vi "Product Romete Exchange.vi"(8 "error in (no error)":errorcluster, 11 "Main":T1={"Tite"="", "Base path"=path "", "Table"=[], "Stations"=[], "Shield Array"=[], "UPHs"=[], "VISA"={"VISA"="", "baud rate"=9600, "data bits"=8, "parity"=enum."None", "stop bits"=10, "flow control"=0}, "Path"={"roof"=path "", "Config"=path "", "Png"=path ""}, "Ctr"={"DB Dispaly"=refnum, "Error Table"=refnum, "Display"=refnum, "Login"=refnum, "Exit"=refnum, "FTT_Submit"=refnum}, "Login"={"User"="", "Grade"=""}, "information"={"cause"="", "Type"=enum."Inform", "code"=0, "Suroce"="", "Status"=FALSE}, "Local DB"={"Connstr"="", "Database"={"Constr"={"Driver"="", "Server"="", "User"="", "Pwd"="", "Database"=""}, "conn ref"=refnum, "State"=FALSE}}, "Remote DB"={"Connstr"="", "Database"={"Constr"={"Driver"="", "Server"="", "User"="", "Pwd"="", "Database"=""}, "conn ref"=refnum, "State"=FALSE}}, "FTT TV"="", "ExchangeTime"=0, "NVH"="", "EOL Path"=path ""} {"VISA"."flow control" items=["None", "XON/XOFF", "RTS/CTS", "XON/XOFF & RTS/CTS", "DTR/DSR", "XON/XOFF & DTR/DSR"]; "VISA"."stop bits" items=["1.0"=10, "1.5"=15, "2.0"=20]}) -> (0 "error out":errorcluster)   [LabVIEW 2014]
uses:
  <vilib>/addons/database/_DB Variant To Data/Database Variant To Data.xnode
  Type'def/AJ_RunTable.ctl
  Type'def/Exchange Table.ctl
  <vilib>/ptbypt/NI_PtbyPt.lvlib
  Simatic S7/Function/Read/Read Sigle Data/Read Sigle String.vi
  <vilib>/addons/database/NI_Database_API.lvlib
  Type'def/BR Exchange(Romte).ctl
  Type'def/Online_Table.ctl
  Simatic S7/Function/Write/Write Sigle Data/Write Sigle Bool.vi
  Type'def/UPH Config.ctl
  VISA/Ctr/VISA Ctr.ctl
  Type'def/Main Ctr Ref.ctl
  Type'def/User Login.ctl
  Database/Ctr/Constr.ctl
  <vilib>/addons/database/Connection.llb/Conn ObjectReference.ctl
  Database/Ctr/Conneect State.ctl
  Type'def/MainCtr.ctl
panel:
  out "Previous Event":string
  in  "Test":bool
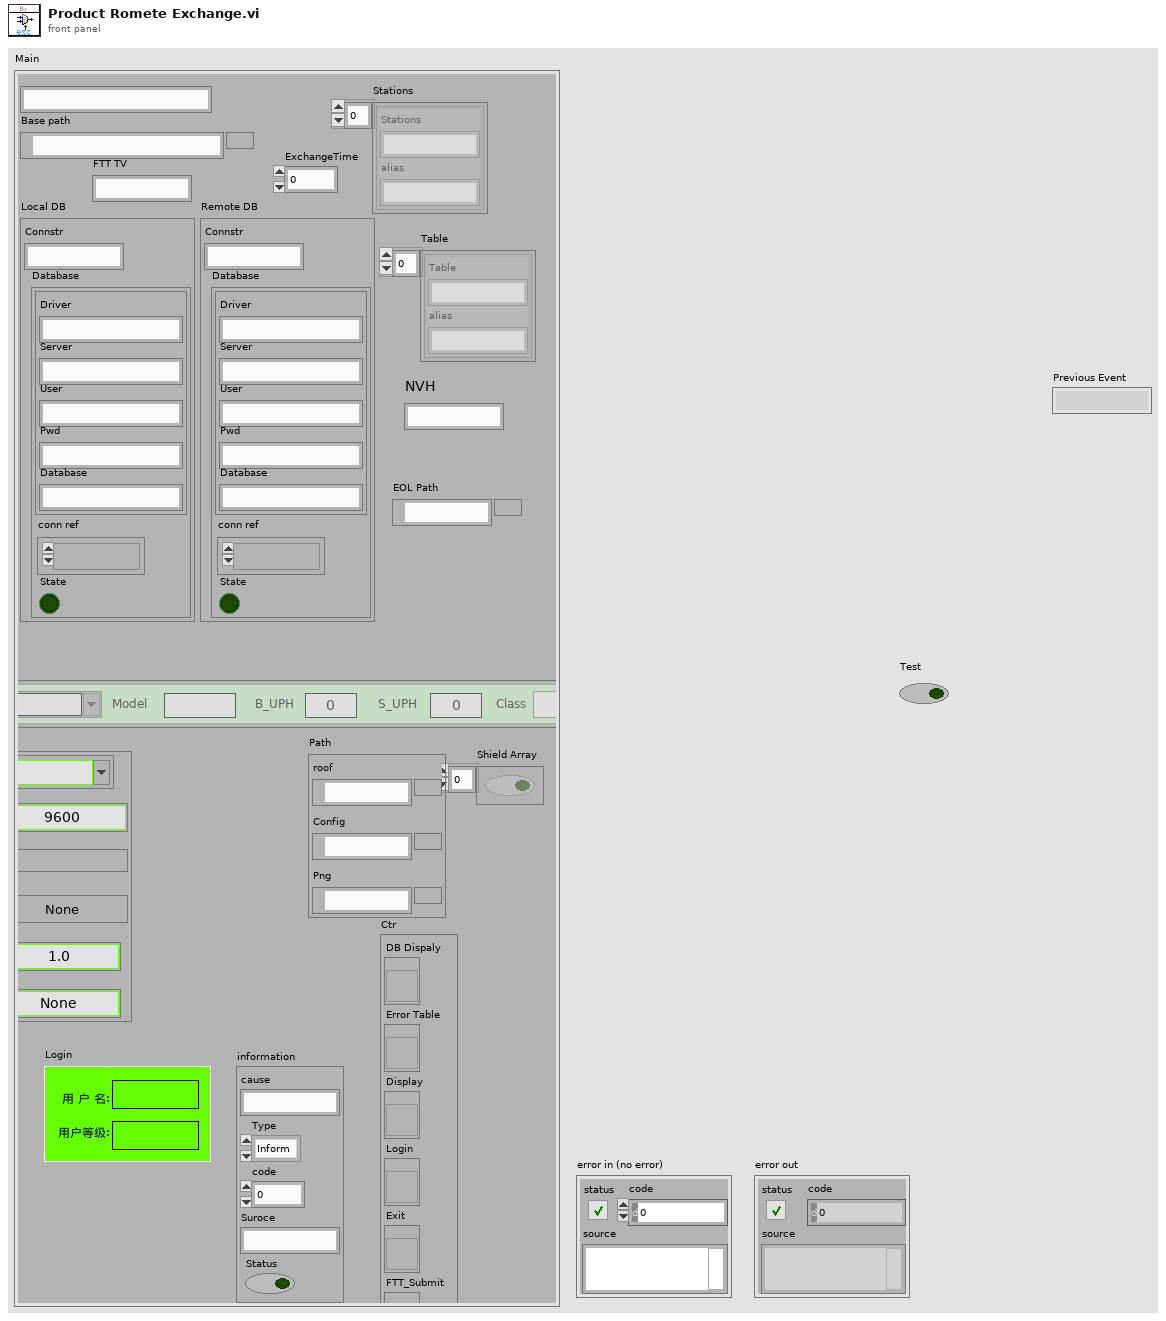
[diagram p1: front panel]
types:
  T1 = typedef "MainCtr.ctl" = cluster{"Tite":string, "Base path":path, "Table":cluster{"Table":string, "alias":string}[], "Stations":cluster{"Stations":string, "alias":string}[], "Shield Array":bool[], "UPHs":T2[], "VISA":T3, "Path":cluster{"roof":path, "Config":path, "Png":path}, "Ctr":T4, "Login":T5, "information":cluster{"cause":string, "Type":enum16{"Inform", "Warning", "Alarm"}, "code":i32, "Suroce":string, "Status":bool}, "Local DB":cluster{"Connstr":string, "Database":T6}, "Remote DB":cluster{"Connstr":string, "Database":T6}, "FTT TV":string, "ExchangeTime":i32, "NVH":string, "EOL Path":path}
  T2 = typedef "UPH Config.ctl" = cluster{"Line_No":string, "Model":string, "B_UPH ":i16, "S_UPH  ":i16, "Class":enum16{"Big", "Small"}}
  T3 = typedef "VISA Ctr.ctl" = cluster{"VISA":refnum<visa-resource-name>, "baud rate":u32, "data bits":u16, "parity":enum16{"None", "Odd", "Even", "Mark", "Space"}, "stop bits":u16, "flow control":u16}
  T4 = typedef "Main Ctr Ref.ctl" = cluster{"DB Dispaly":refnum<vi>, "Error Table":refnum<vi>, "Display":refnum<vi>, "Login":refnum<vi>, "Exit":refnum<vi>, "FTT_Submit":refnum<vi>}
  T5 = typedef "User Login.ctl" = cluster{"User":string, "Grade":string}
  T6 = typedef "Conneect State.ctl" = cluster{"Constr":T7, "conn ref":T8, "State":bool}
  T7 = typedef "Constr.ctl" = cluster{"Driver":string, "Server":string, "User":string, "Pwd":string, "Database":string}
  T8 = typedef "NI_Database_API.lvlib/Conn ObjectReference.ctl" = refnum<k1>
  T9 = cluster{"Next PN":cluster{"SN":string, "Model":string, "Pos":i32}, "PrePN":cluster{"SN":string, "Model":string, "Pos":i32}}
  T10 = typedef "Exchange Table.ctl" = cluster{"LineName":string, "Model":string, "Station":string, "StartTime":timestamp, "EndTime":timestamp, "SubTime":dbl}
  T11 = typedef "AJ_RunTable.ctl" = cluster{"LineName":string, "ProjectName":string, "AcutalOuput":u32, "ProStatus":string, "PlanOutput":u32, "ProTime":u32, "ShiftFlag":string}
  T12 = cluster{"cause":string, "Type":enum16{"Inform", "Warning", "Alarm"}, "code":i32, "Suroce":string, "Status":bool}
  T13 = typedef "BR Exchange(Romte).ctl" = cluster{"Line Name":string, "Start Tine":timestamp, "End Time":timestamp, "PrePN":string, "NextPN":string, "Status":bool}
  T14 = cluster{"excT":dbl, "Pos":cluster{"Pre Pos":i32, "Next Pos":i32}, "relative s":dbl, "Exchange Table":T10, "Main ":T1, "BR":T13, "information":cluster{"cause":string, "Type":enum16{"Inform", "Warning", "Alarm"}, "code":i32, "Suroce":string, "Status":bool}, "UPH Model":string[], "FTT Log":string[], "AJ Run":T11, "Exc flag":cluster{"Exchange Enable":bool, "ms":dbl}, "ExcPN":cluster{"Next PN":cluster{"SN":string, "Model":string, "Pos":i32}, "PrePN":cluster{"SN":string, "Model":string, "Pos":i32}}}
  T15 = typedef "Online_Table.ctl" = cluster{"SN":string, "Frame":string, "Station":string, "Model":string, "Color":string, "OnTime":timestamp, "OutTime":timestamp, "Repaired":i32, "OnRepair":bool, "Pstate":string}
  T16 = cluster{"Array str[0]":string, "Array str[1]":string, "Array str[2]":string, "Array str[3]":string, "Array str[4]":string, "Array str[5]":string, "Array str[6]":string, "Array str[7]":string, "Array str[8]":string, "Array str[9]":string, "Array str[10]":string}
  T17 = typedef "FTT Display Type.ctl" = cluster{"Line.No":string, "Model":string, "Color":string, "UPH":dbl, "Plan":dbl, "Target Rate":dbl, "Target ":dbl, "Actual":dbl, "FTT":dbl, "FTT Rate":dbl, "Repaired":dbl, "Reject":dbl, "Ouline":dbl, "Line State":string}
  T18 = cluster{"Display":T17, "Class":enum16{"Big", "Small"}}
  T19 = typedef "Phone Var.ctl" = cluster{"Mes":bool, "Model":string}
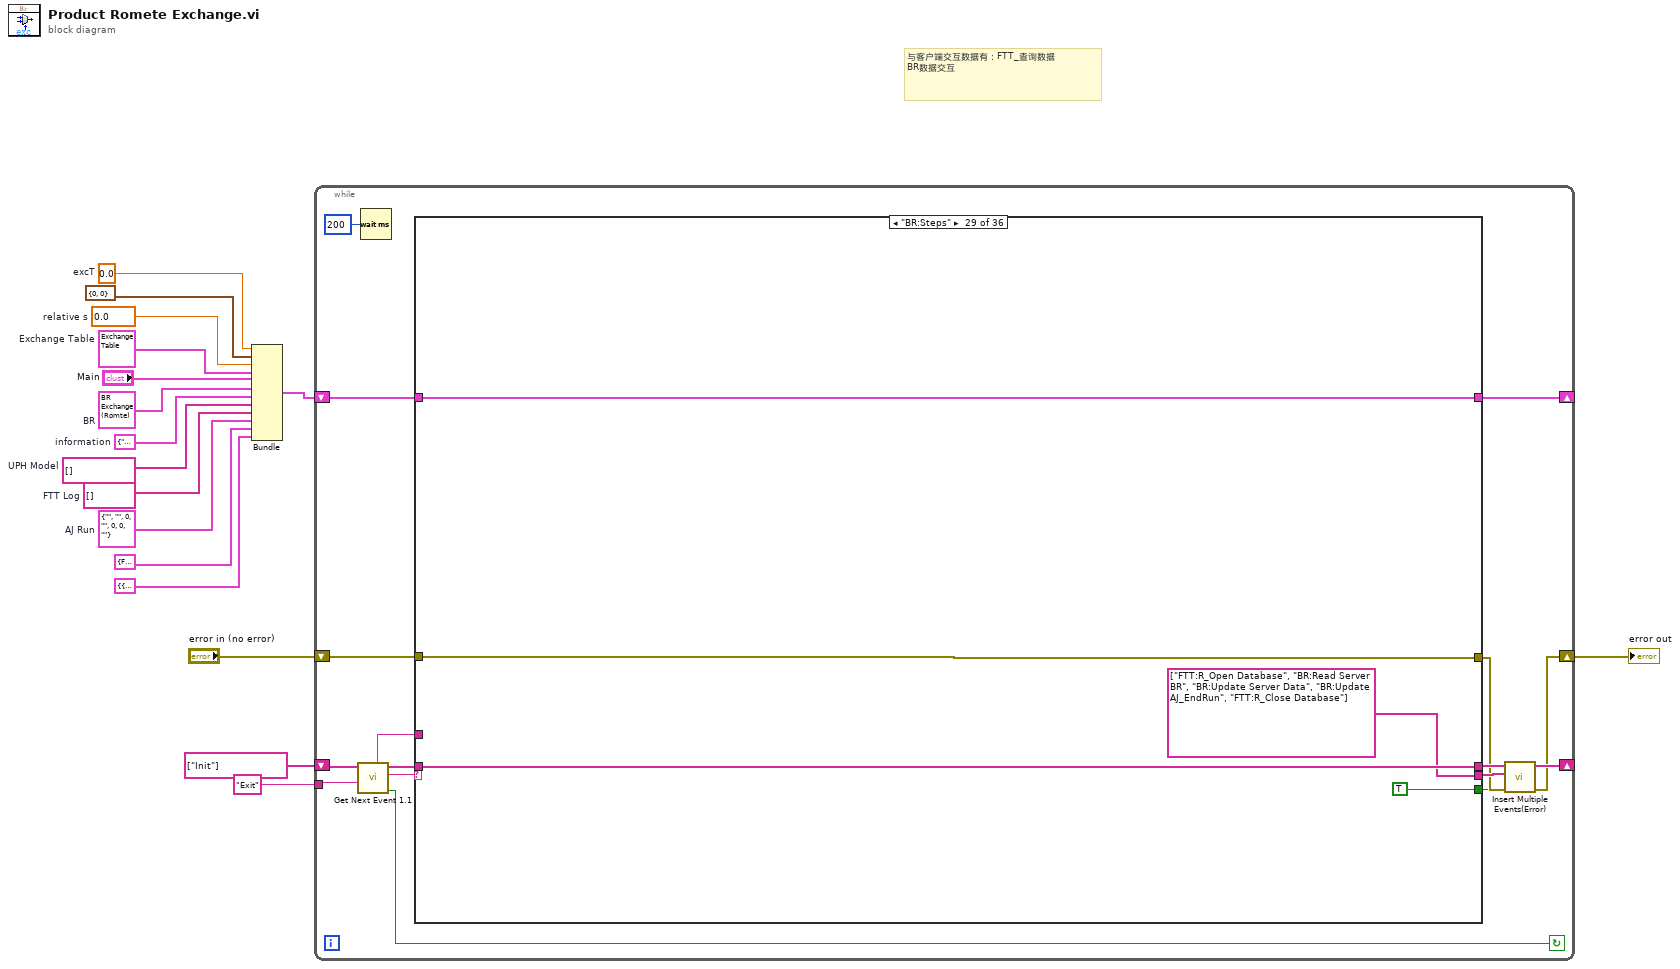
[diagram p0: block diagram]
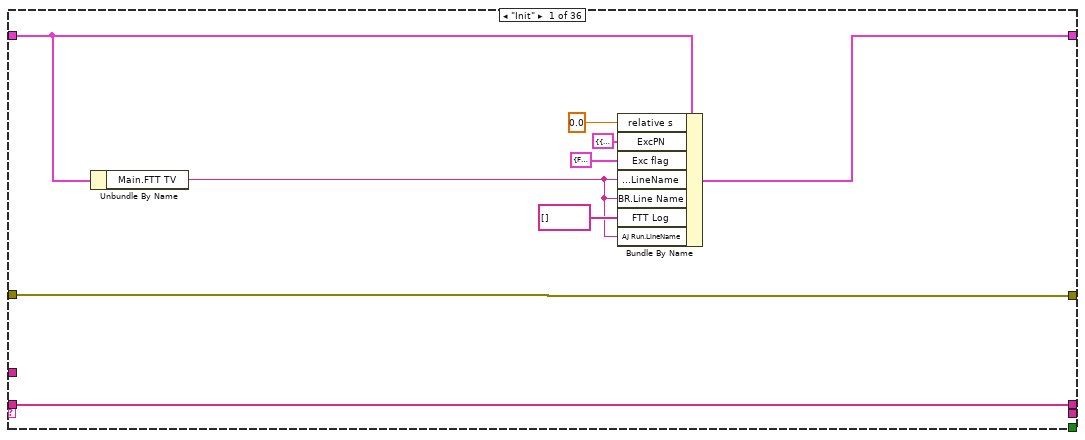
[diagram p2: hidden frame]
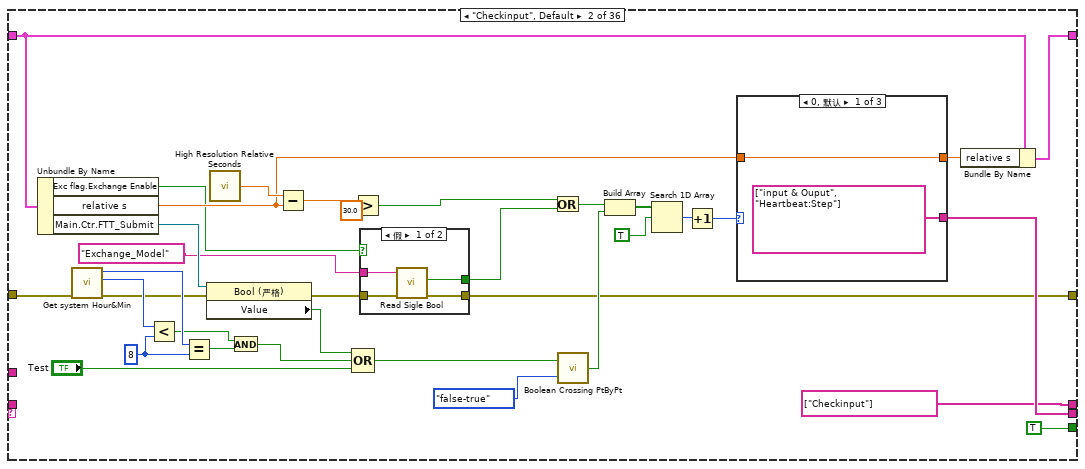
[diagram p3: hidden frame]
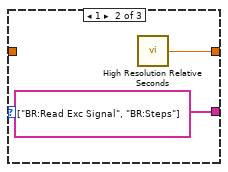
[diagram p5: hidden frame]
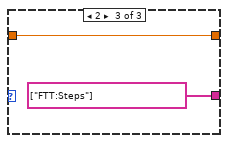
[diagram p6: hidden frame]
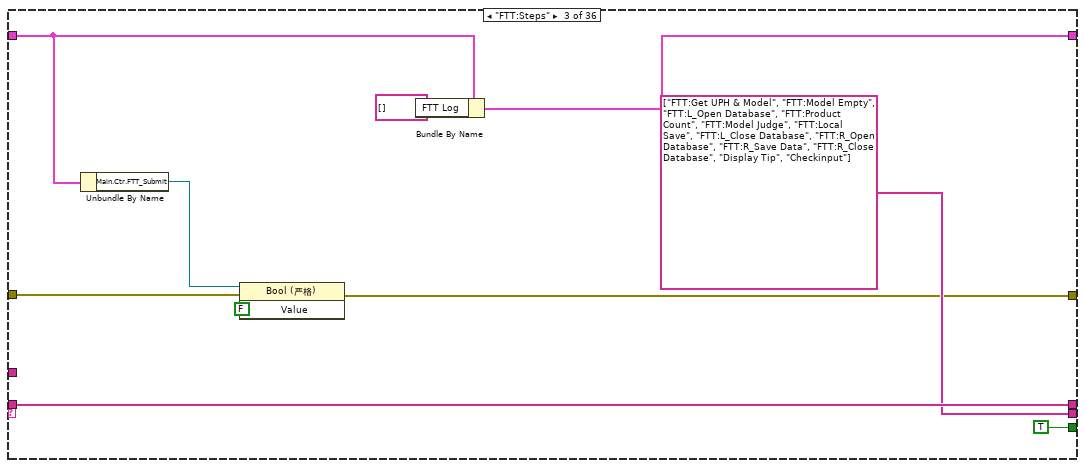
[diagram p7: hidden frame]
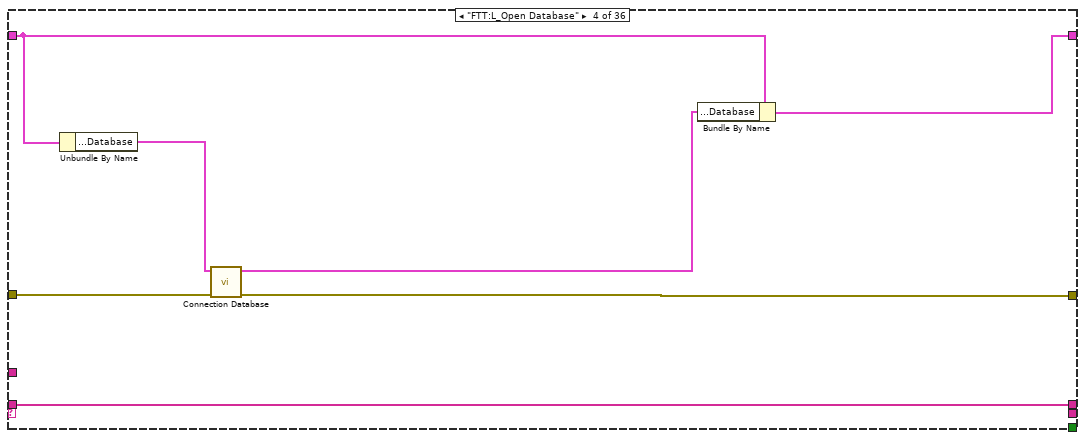
[diagram p8: hidden frame]
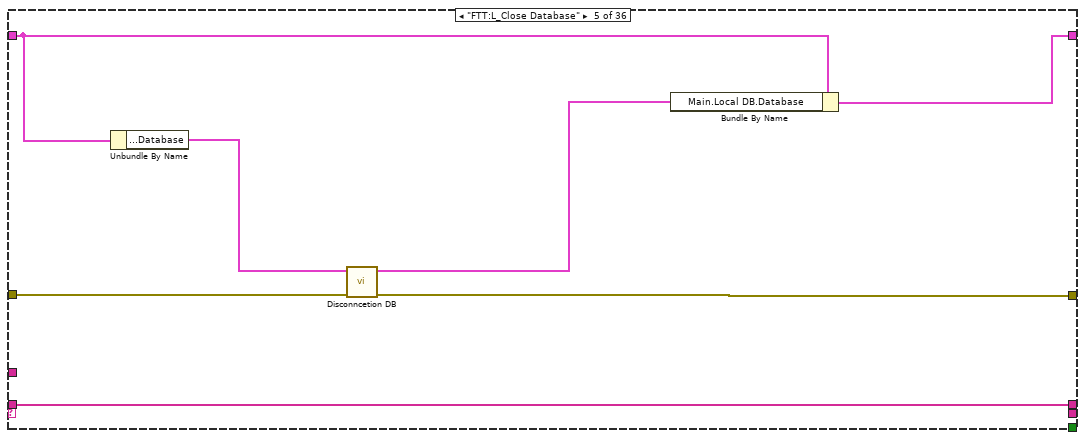
[diagram p9: hidden frame]
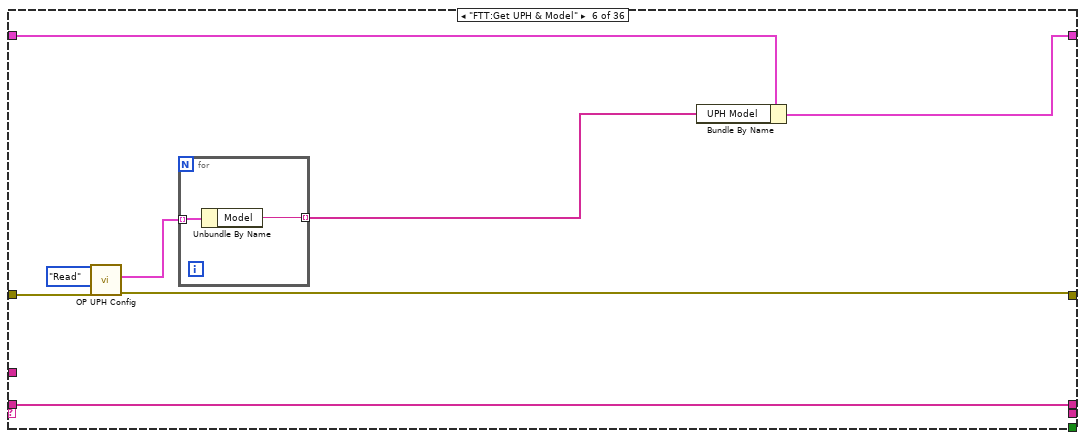
[diagram p10: hidden frame]
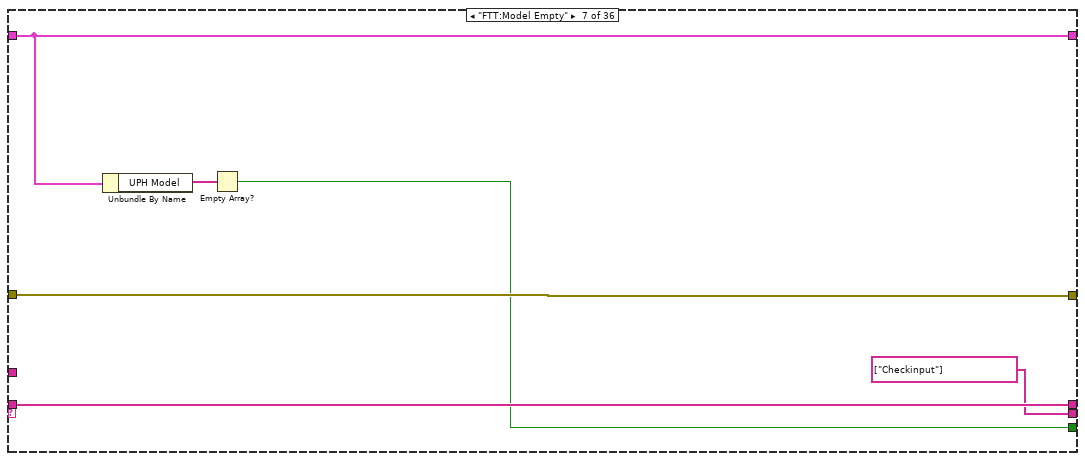
[diagram p11: hidden frame]
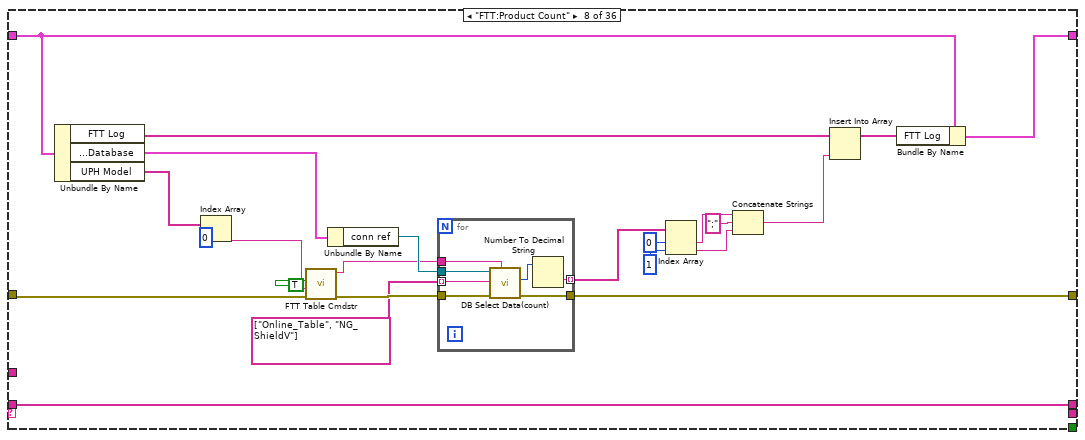
[diagram p12: hidden frame]
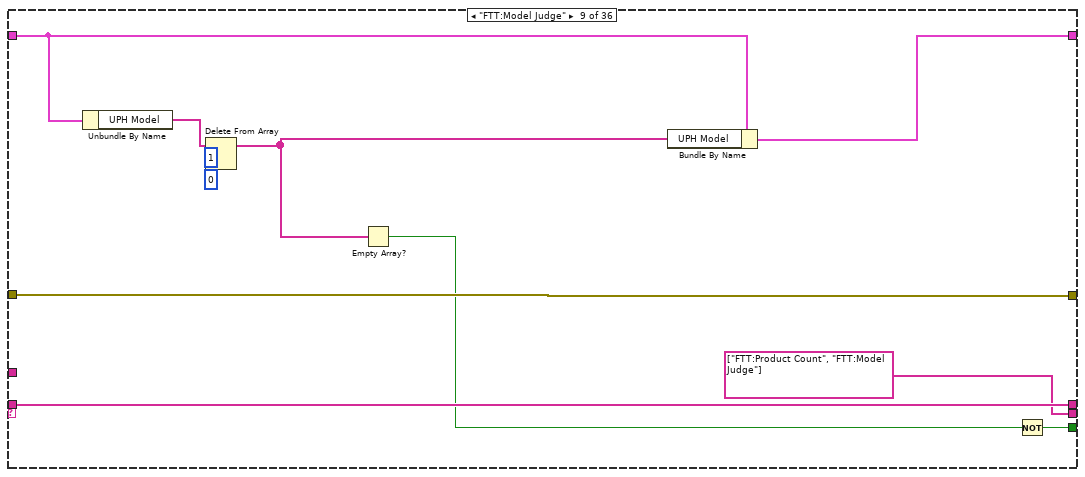
[diagram p13: hidden frame]
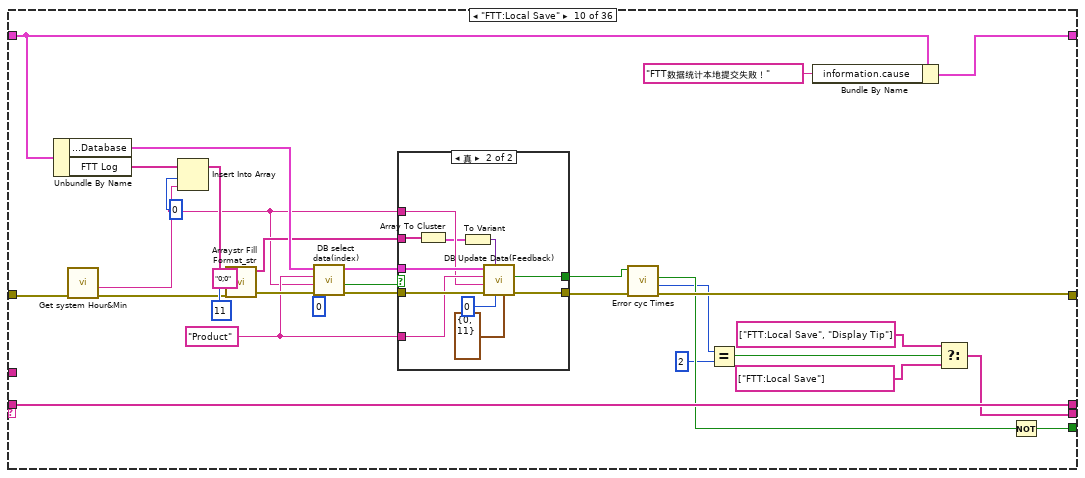
[diagram p14: hidden frame]
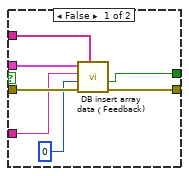
[diagram p15: hidden frame]
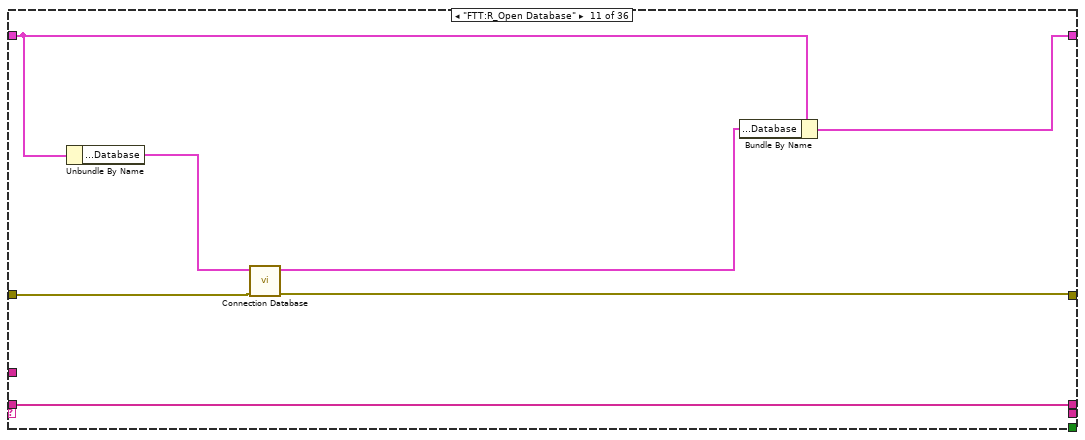
[diagram p16: hidden frame]
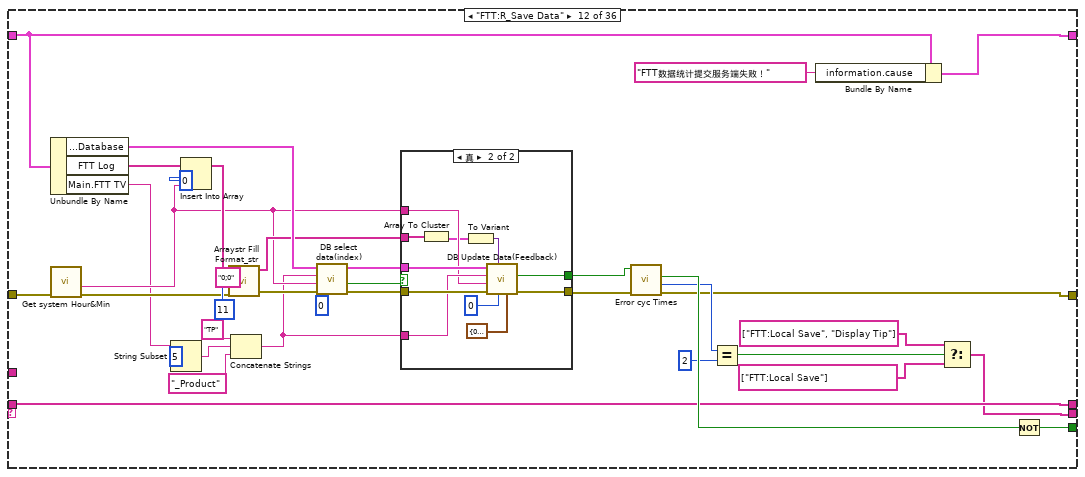
[diagram p17: hidden frame]
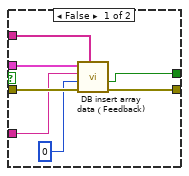
[diagram p18: hidden frame]
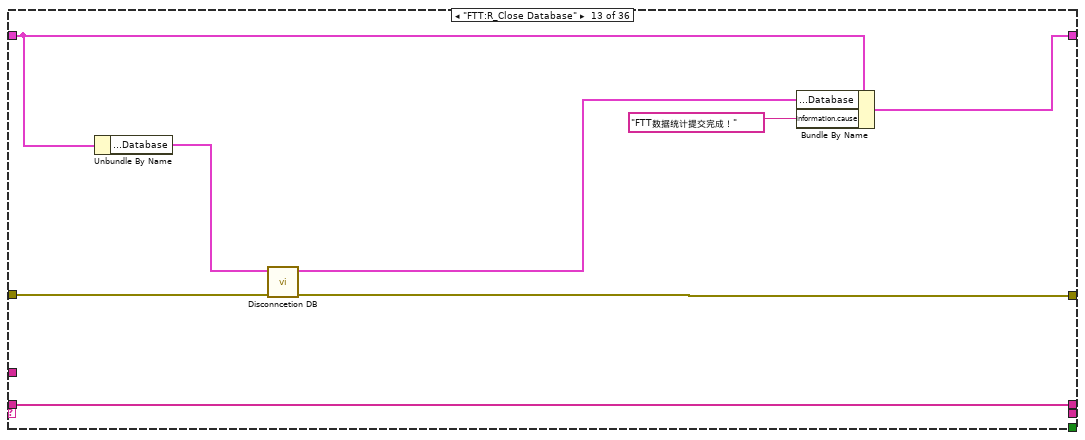
[diagram p19: hidden frame]
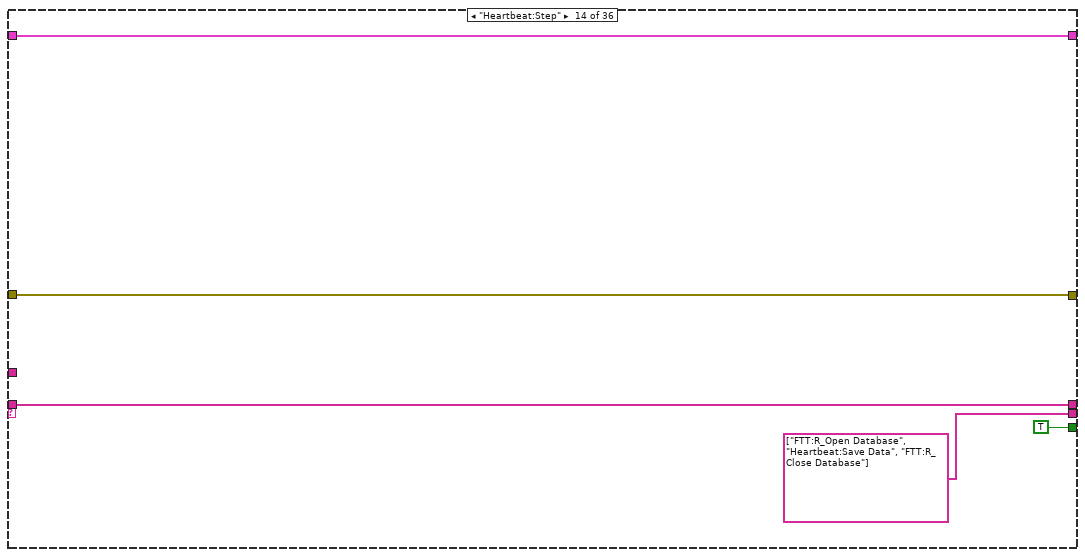
[diagram p20: hidden frame]
diagram:
  w1 = 0.0  # excT
  w3 = 0.0  # relative s
  w6 = T10 {"LineName"="", "Model"="", "Station"="", "StartTime"=timestamp(0 s since 1904-01-01), "EndTime"=timestamp(0 s since 1904-01-01), "SubTime"=0.0}  # Exchange Table
  w7 = T11 {"LineName"="", "ProjectName"="", "AcutalOuput"=0, "ProStatus"="", "PlanOutput"=0, "ProTime"=0, "ShiftFlag"=""}  # AJ Run
  w8 = string[] []  # FTT Log
  w9 = string[] []  # UPH Model
  w10 = T12 {"cause"="", "Type"=enum."Inform", "code"=0, "Suroce"="", "Status"=FALSE}  # information
  w12 = T13 {"Line Name"="", "Start Tine"=timestamp(0 s since 1904-01-01), "End Time"=timestamp(0 s since 1904-01-01), "PrePN"="", "NextPN"="", "Status"=FALSE}  # BR
  # "与客户端交互数据有：FTT_查询数据\nBR数据交互"
  n1 = Bundle("excT"=w1, "Pos"=cluster{"Pre Pos":i32, "Next Pos":i32} {"Pre Pos"=0, "Next Pos"=0}, "relative s"=w3, "Exchange Table"=w6, "Main"="Main", "BR"=w12, "information"=w10, "UPH Model"=w9, "FTT Log"=w8, "AJ Run"=w7, "Exc flag"=cluster{"Exchange Enable":bool, "ms":dbl} {"Exchange Enable"=FALSE, "ms"=0.0}, "ExcPN"=T9 {"Next PN"={"SN"="", "Model"="", "Pos"=0}, "PrePN"={"SN"="", "Model"="", "Pos"=0}}) -> (w14:T14)  [unwired: 1 in]
  n2 = while {
    tunnel: "Exit" ("Exit Event") -> [w30]
    shift-right: [w26] -> _
    shift-left: string[] ["Init"] -> [w31]
    shift-right: [w21] -> w11
    shift-left: "error in (no error)" -> [w29]
    shift-right: [w23] -> _
    shift-left: w14 -> [w27]
    stop <- w32 continue-if-true
    n3 = call "Get Next Event 1.1.vi"("Exit Event"=w30, "event queue in"=w31) -> ("Condition (Exit:F)"=w32:bool, "next event"=w33:string, "event queue out"=w28:string[], "Previous Event"=w18:string)  [unwired: 6 in]
    n4 = Wait (ms)(milliseconds to wait=u32 200) -> ()  [unwired: 1 out]
    n5 = case shown="\"BR:Steps\"" w33 {
      tunnel: w29 -> [w41 w76 w95 w105 w111 w120 w126 w151 w166 w195 w225 w233 w286 w291 w317 w354 w359 w364 w377 w404 w457 w860 w919 w983 w1254 w1305 w1712 w2017 w2066 w2079 w2343 w2399 w2468 w2474 w2479 w2490]
      tunnel: w28 -> [w42 _ w98 w104 w112 w113 w125 w140 w165 w179 w224 w238 w287 w290 w314 w355 w358 w362 w374 w403 w458 w861 w920 w979 w1255 w1277 w1706 w2006 w2065 w2069 w2338 w2404 w2464 w2470 w2478 _]
      tunnel: w27 -> [w36 w55 w90 w102 w108 w116 w128 w130 w160 w181 w221 w234 w284 w292 w295 w348 w360 w367 w370 w401 w455 w853 w903 w959 w1243 w1286 w1701 w1997 w2067 w2072 w2325 w2403 w2466 w2475 w2480 w2487]
      tunnel: [w41 w46 w93 w99 w109 w118 w126 w141 w166 w182 w222 w235 w282 w291 w304 w353 w359 w364 w375 w399 w456 w859 w900 w969 w1250 w1288 w1702 w1994 w2066 w2070 w2334 w2402 w2467 w2472 w2479 w2488] -> w22
      tunnel: [w42 string[] ["Checkinput"] w98 w104 w112 w113 w125 w140 w165 w179 w224 w238 w287 w290 w314 w355 w358 w362 w374 w403 w458 w861 w920 w979 w1255 w1277 w1706 w2006 w2065 w2069 w2338 w2404 w2464 w2470 w2478 string[] ["Checkinput"]] -> w25
      tunnel: [_ TRUE ("Insert all? (T)") TRUE ("Insert all? (T)") _ _ _ w124 _ w164 w178 _ w236 _ TRUE ("Insert all? (T)") w303 TRUE ("Insert all? (T)") TRUE ("Insert all? (T)") w363 _ _ _ _ w910 w965 w1244 _ w1698 w2005 TRUE ("Insert all? (T)") _ w2333 w2401 _ w2471 TRUE ("Insert all? (T)") FALSE ("Insert all? (T)")] -> w20
      tunnel: [_ w68 string[] ["FTT:Get UPH & Model", "FTT:Model Empty", "FTT:L_Open Database", "FTT:Product Count", "FTT:Model Judge", "FTT:Local Save", "FTT:L_Close Database", "FTT:R_Open Database", "FTT:R_Save Data", "FTT:R_Close Database", "Display Tip", "Checkinput"] _ _ _ string[] ["Checkinput"] _ string[] ["FTT:Product Count", "FTT:Model Judge"] w172 _ w237 _ string[] ["FTT:R_Open Database", "Heartbeat:Save Data", "FTT:R_Close Database"] w298 w342 string[] ["FTT:L_Open Database", "Exchange:Init Steps", "Exchange:Get Next SN", "Exchange:Serch SN Pos", "Exchange:Exc PrePN Table", "Exchange:Exc NextPN Table Update", "Exchange:End Judge", "FTT:L_Close Database"] string[] ["Exchange:Ready ok", "Exchange:Reset Exc Signal", "Display Tip"] _ _ _ _ w906 w972 string[] ["Exchange:Read OutTime", "Exchange:Get Esc SubTimeMax", "Display Tip"] _ string[] ["Display Tip", "FTT:R_Open Database", "Exchange:Server_exc Table", "FTT:R_Close Database"] w2000 string[] ["FTT:R_Open Database", "BR:Read Server BR", "BR:Update Server Data", "BR:Update AJ_EndRun", "FTT:R_Close Database"] _ w2326 w2400 _ string[] ["Quit"] string[] ["Exit"] _] -> w24
      tunnel: [w39 w54 w89 w101 w106 w115 w128 w129 w159 w180 w220 w232 w283 w292 w294 w347 w360 w367 w369 w400 w454 w852 w902 w958 w1243 w1285 w1700 w1996 w2067 w2071 w2325 w2403 w2466 w2475 w2480 w2487] -> w23
      tunnel: w18 -> [_ _ _ _ _ _ _ _ _ _ _ _ _ _ _ _ _ _ _ _ _ _ _ _ _ _ _ _ _ _ _ _ _ _ _ w2482]
      frame "Init" {
        n6 = Unbundle By Name(w36) -> ("Main.FTT TV"=w34:string)
        n7 = Bundle By Name(cluster=w36, "relative s"=0.0, "ExcPN"=T9 {"Next PN"={"SN"="", "Model"="", "Pos"=0}, "PrePN"={"SN"="", "Model"="", "Pos"=0}}, "Exc flag"=cluster{"Exchange Enable":bool, "ms":dbl} {"Exchange Enable"=FALSE, "ms"=0.0}, "Exchange Table.LineName"=w34, "BR.Line Name"=w34, "FTT Log"=string[] [], "AJ Run.LineName"=w34) -> (w39:T14)
      }
      frame "Checkinput", Default {
        w73 = 8 ("hour")
        n8 = Unbundle By Name(w55) -> ("Exc flag.Exchange Enable"=w48:bool, "relative s"=w53:dbl, "Main.Ctr.FTT_Submit"=w65:refnum<vi>)
        n9 = call "Get system Hour&Min.vi"("error in (no error)"=w76) -> ("error out"=w66:errorcluster, "minute"=w74:i32, "hour"=w75:i32)  [unwired: 7 in, 1 out]
        n10 = Less?(x=w74, y=w73) -> (x < y?=w71:bool)
        n11 = Equal?(x=w75, y=w73) -> (x = y?=w72:bool)
        n12 = property class="Bool (严格)"(reference=w65, error in=w66) -> (error out=w49:errorcluster, "Value"=w64:bool)  [unwired: 1 out]
        n13 = call <vilib>:"High Resolution Relative Seconds.vi"() -> ("relative seconds"=w63:dbl)
        n14 = And(x=w71, y=w72) -> (x .and. y?=w69:bool)
        n15 = Subtract(x=w63, y=w53) -> (x-y=w62:dbl)
        n16 = Compound Arithmetic op=OR(w64, w69, "Test") -> (w51:bool)
        n17 = Greater?(x=w62, y=30.0) -> (0:w44:bool)
        n18 = case shown="假" w48 {
          tunnel: w49 -> [w81 w82]
          tunnel: "Exchange_Model" ("Tags") -> [w80 _]
          tunnel: [w79 w82] -> w46
          tunnel: [w78 _] -> w43
          frame False {
            n19 = call "Read Sigle Bool.vi"("error in (no error)"=w81, "Tags"=w80) -> ("error out"=w79:errorcluster, "Boolean"=w78:bool)  [unwired: 7 in, 1 out]
          }
          frame True {
          }
        }
        n20 = Or(x=w44, y=w43) -> (x .or. y?=w45:bool)
        n21 = call <vilib>:"Boolean Crossing PtByPt.vi"("direction"=enum16{"either", "false-true", "true-false"}."false-true", "input"=w51) -> ("crossing"=w52:bool)  [unwired: 1 in]
        n22 = Build Array(w45, w52) -> (w60:bool[])
        n23 = Search 1D Array(1D array=w60, element=TRUE) -> (index of element=w58:i32)  [unwired: 1 in]
        n24 = Increment(x=w58) -> (x+1=w57:i32)
        n25 = case shown="0, 默认" w57 {
          tunnel: [string[] ["input & Ouput", "Heartbeat:Step"] string[] ["BR:Read Exc Signal", "BR:Steps"] string[] ["FTT:Steps"]] -> w68
          tunnel: [w83 w86 w87] -> w56
          tunnel: w53 -> [w83 _ w87]
          frame 0, Default {
          }
          frame 1 {
            n26 = call <vilib>:"High Resolution Relative Seconds.vi"() -> ("relative seconds"=w86:dbl)
          }
          frame 2 {
          }
        }
        n27 = Bundle By Name(cluster=w55, "relative s"=w56) -> (w54:T14)
      }
      frame "FTT:Steps" {
        n28 = Unbundle By Name(w90) -> ("Main.Ctr.FTT_Submit"=w94:refnum<vi>)
        n29 = property class="Bool (严格)"(reference=w94, error in=w95, "Value"=FALSE) -> (error out=w93:errorcluster)  [unwired: 1 out]
        n30 = Bundle By Name(cluster=w90, "FTT Log"=string[] []) -> (w89:T14)
      }
      frame "FTT:L_Open Database" {
        n31 = Unbundle By Name(w102) -> ("Main.Local DB.Database"=w103:T6)
        n32 = call "Connection Database.vi"("error in (no error)"=w105, "Connncet State"=w103) -> ("error out"=w99:errorcluster, "Connncet State out"=w100:T6)  [unwired: 8 in]
        n33 = Bundle By Name(cluster=w102, "Main.Local DB.Database"=w100) -> (w101:T14)
      }
      frame "FTT:L_Close Database" {
        n34 = Unbundle By Name(w108) -> ("Main.Local DB.Database"=w110:T6)
        n35 = call "Disconncetion DB.vi"("error in (no error)"=w111, "Connncet State"=w110) -> ("error out"=w109:errorcluster, "Connect State"=w107:T6)  [unwired: 8 in]
        n36 = Bundle By Name(cluster=w108, "Main.Local DB.Database"=w107) -> (w106:T14)
      }
      frame "FTT:Get UPH & Model" {
        n37 = call "OP UPH Config.vi"("error in (no error)"=w120, "Enum"=enum16{"init", "Read", "Write"}."Read") -> ("error out"=w118:errorcluster, "UPH out"=w117:T2[])  [unwired: 7 in, 1 out]
        n38 = for {
          tunnel: w117 -> [w122] mode=indexing
          tunnel: [w121] -> w114 mode=indexing
          n39 = Unbundle By Name(w122) -> ("Model"=w121:string)
        }
        n40 = Bundle By Name(cluster=w116, "UPH Model"=w114) -> (w115:T14)
      }
      frame "FTT:Model Empty" {
        n41 = Unbundle By Name(w128) -> ("UPH Model"=w127:string[])
        n42 = Empty Array?(array=w127) -> (empty?=w124:bool)
      }
      frame "FTT:Product Count" {
        n43 = Unbundle By Name(w130) -> ("FTT Log"=w133:string[], "Main.Local DB.Database"=w145:T6, "UPH Model"=w149:string[])
        n44 = Index Array(array=w149, index=0) -> (element=w148:string)
        n45 = call "FTT Table Cmdstr.vi"("error in (no error)"=w151, "Model"=w148, "Pstate"=TRUE) -> ("error out"=w146:errorcluster, "Str"=w143:string)  [unwired: 7 in]
        n46 = Unbundle By Name(w145) -> ("conn ref"=w144:T8)
        n47 = for {
          tunnel: w146 -> [w158]
          tunnel: w144 -> [w157]
          tunnel: w143 -> [w156]
          tunnel: string[] ["Online_Table", "NG_ShieldV"] -> [w155] mode=indexing
          tunnel: [w154] -> w141
          tunnel: [w152] -> w139 mode=indexing
          n48 = call "DB Select Data(count).vi"("condition"=w156, "error in (no error)"=w158, "table"=w155, "connection reference"=w157) -> ("error out"=w154:errorcluster, "Count"=w153:i32)  [unwired: 5 in, 1 out]
          n49 = Number To Decimal String(number=w153) -> (decimal integer string=w152:string)  [unwired: 1 in]
        }
        n50 = Index Array(array=w139, index #1=0 ("index"), index #2=1 ("index")) -> (element #1=w136:string, element #2=w134:string)
        n51 = Concatenate Strings(w136, ";" ("string"), w134) -> (w132:string)
        n52 = Insert Into Array(array=w133, new element=w132) -> (w131:string[])  [unwired: 1 in]
        n53 = Bundle By Name(cluster=w130, "FTT Log"=w131) -> (w129:T14)
      }
      frame "FTT:Model Judge" {
        n54 = Unbundle By Name(w160) -> ("UPH Model"=w169:string[])
        n55 = Delete From Array(array=w169, length=1, index=0) -> (array with subset deleted=w161:string[])  [unwired: 1 out]
        n56 = Empty Array?(array=w161) -> (empty?=w163:bool)
        n57 = Bundle By Name(cluster=w160, "UPH Model"=w161) -> (w159:T14)
        n58 = Not(x=w163) -> (.not. x?=w164:bool)
      }
      frame "FTT:Local Save" {
        w186 = "Product" ("table")
        n59 = Unbundle By Name(w181) -> ("Main.Local DB.Database"=w197:T6, "FTT Log"=w193:string[])
        n60 = call "Get system Hour&Min.vi"("error in (no error)"=w195) -> ("error out"=w194:errorcluster, "date/time string"=w185:string)  [unwired: 7 in, 2 out]
        n61 = Insert Into Array(array=w193, index=0, new element=w185) -> (w192:string[])
        n62 = call "Arraystr Fill Format_str.vi"("error in (no error)"=w194, "Len"=u32 11, "Format_str"="0;0", "Array"=w192) -> ("error out"=w198:errorcluster, "Array str"=w188:string[])  [unwired: 6 in]
        n63 = call "DB select data(index).vi"("index"=0, "error in (no error)"=w198, "Code"=w185, "Tabe"=w186, "Connncet State"=w197) -> ("error out"=w190:errorcluster, "state"=w189:bool, "Connncet State out"=w187:T6)  [unwired: 3 in, 1 out]
        n64 = case shown="真" w189 {
          tunnel: w190 -> [w207 w218]
          tunnel: w188 -> [w206 w212]
          tunnel: w187 -> [w205 w217]
          tunnel: w186 -> [w204 w216]
          tunnel: w185 -> [_ w215]
          tunnel: [w202 w213] -> w184
          tunnel: [w201 w209] -> w183
          frame False {
            n65 = call "DB insert array data（Feedback).vi"("Data"=w206, "error in (no error)"=w207, "index"=0, "table"=w204, "Connncet State"=w205) -> ("error out"=w202:errorcluster, "state"=w201:bool)  [unwired: 4 in, 1 out]
          }
          frame True {
            n66 = Array To Cluster(array=w212) -> (cluster=w211:T16)
            n67 = To Variant(anything=w211) -> (Variant=w210:variant)
            n68 = call "DB Update Data(Feedback).vi"("Pos"=cluster{"index":i32, "Len":i32} {"index"=0, "Len"=11}, "Sel index"=0, "data"=w210, "error in (no error)"=w218, "Code"=w215, "table"=w216, "Connncet State"=w217) -> ("error out"=w213:errorcluster, "State"=w209:bool)  [unwired: 2 in, 1 out]
          }
        }
        n69 = call "Error cyc Times.vi"("error in (no error)"=w184, "Status in"=w183) -> ("error out"=w182:errorcluster, "Numeric"=w176:i32, "Cys Status"=w177:bool)  [unwired: 6 in, 1 out]
        n70 = Equal?(x=w176, y=2) -> (x = y?=w174:bool)
        n71 = Bundle By Name(cluster=w181, "information.cause"="FTT数据统计本地提交失败！") -> (w180:T14)
        n72 = Select(t=string[] ["FTT:Local Save", "Display Tip"], s=w174, f=string[] ["FTT:Local Save"]) -> (s? t:f=w172:string[])
        n73 = Not(x=w177) -> (.not. x?=w178:bool)
      }
      frame "FTT:R_Open Database" {
        n74 = Unbundle By Name(w221) -> ("Main.Remote DB.Database"=w223:T6)
        n75 = call "Connection Database.vi"("error in (no error)"=w225, "Connncet State"=w223) -> ("error out"=w222:errorcluster, "Connncet State out"=w219:T6)  [unwired: 8 in]
        n76 = Bundle By Name(cluster=w221, "Main.Remote DB.Database"=w219) -> (w220:T14)
      }
      frame "FTT:R_Save Data" {
        n77 = Unbundle By Name(w234) -> ("Main.Remote DB.Database"=w258:T6, "FTT Log"=w255:string[], "Main.FTT TV"=w231:string)
        n78 = call "Get system Hour&Min.vi"("error in (no error)"=w233) -> ("error out"=w256:errorcluster, "date/time string"=w248:string)  [unwired: 7 in, 2 out]
        n79 = String Subset(string=w231, offset (0)=5) -> (substring=w228:string)  [unwired: 1 in]
        n80 = Insert Into Array(array=w255, index=0, new element=w248) -> (w254:string[])
        n81 = call "Arraystr Fill Format_str.vi"("error in (no error)"=w256, "Len"=u32 11, "Format_str"="0;0", "Array"=w254) -> ("error out"=w259:errorcluster, "Array str"=w250:string[])  [unwired: 6 in]
        n82 = Concatenate Strings("TP", w228, "_Product" ("table")) -> (w226:string)
        n83 = call "DB select data(index).vi"("index"=0, "error in (no error)"=w259, "Code"=w248, "Tabe"=w226, "Connncet State"=w258) -> ("error out"=w252:errorcluster, "state"=w251:bool, "Connncet State out"=w249:T6)  [unwired: 3 in, 1 out]
        n84 = case shown="真" w251 {
          tunnel: w252 -> [w268 w279]
          tunnel: w250 -> [w267 w273]
          tunnel: w249 -> [w266 w278]
          tunnel: w226 -> [w265 w277]
          tunnel: w248 -> [_ w276]
          tunnel: [w263 w274] -> w247
          tunnel: [w262 w270] -> w246
          frame False {
            n85 = call "DB insert array data（Feedback).vi"("Data"=w267, "error in (no error)"=w268, "index"=0, "table"=w265, "Connncet State"=w266) -> ("error out"=w263:errorcluster, "state"=w262:bool)  [unwired: 4 in, 1 out]
          }
          frame True {
            n86 = Array To Cluster(array=w273) -> (cluster=w272:T16)
            n87 = To Variant(anything=w272) -> (Variant=w271:variant)
            n88 = call "DB Update Data(Feedback).vi"("Pos"=cluster{"index":i32, "Len":i32} {"index"=0, "Len"=11}, "Sel index"=0, "data"=w271, "error in (no error)"=w279, "Code"=w276, "table"=w277, "Connncet State"=w278) -> ("error out"=w274:errorcluster, "State"=w270:bool)  [unwired: 2 in, 1 out]
          }
        }
        n89 = call "Error cyc Times.vi"("error in (no error)"=w247, "Status in"=w246) -> ("error out"=w235:errorcluster, "Numeric"=w244:i32, "Cys Status"=w245:bool)  [unwired: 6 in, 1 out]
        n90 = Equal?(x=w244, y=2) -> (x = y?=w242:bool)
        n91 = Bundle By Name(cluster=w234, "information.cause"="FTT数据统计提交服务端失败！") -> (w232:T14)
        n92 = Select(t=string[] ["FTT:Local Save", "Display Tip"], s=w242, f=string[] ["FTT:Local Save"]) -> (s? t:f=w237:string[])
        n93 = Not(x=w245) -> (.not. x?=w236:bool)
      }
      frame "FTT:R_Close Database" {
        n94 = Unbundle By Name(w284) -> ("Main.Remote DB.Database"=w285:T6)
        n95 = call "Disconncetion DB.vi"("error in (no error)"=w286, "Connncet State"=w285) -> ("error out"=w282:errorcluster, "Connect State"=w281:T6)  [unwired: 8 in]
        n96 = Bundle By Name(cluster=w284, "Main.Remote DB.Database"=w281, "information.cause"="FTT数据统计提交完成！") -> (w283:T14)
      }
      frame "Heartbeat:Step" {
      }
      frame "Heartbeat:Save Data" {
        w309 = "HeartBeat"
        n97 = Unbundle By Name(w295) -> ("Main.Remote DB.Database"=w316:T6, "Main.FTT TV"=w308:string)
        n98 = String Subset(string=w308, offset (0)=5) -> (substring=w320:string)  [unwired: 1 in]
        n99 = Format Date/Time String(time format string (%c)="%D%M%S") -> (date/time string=w310:string)  [unwired: 2 in]
        n100 = Build Array(w308, w320, w310) -> (w307:string[])
        n101 = call "DB Select data(Count index).vi"("index"=0, "error in (no error)"=w317, "Code"=w308, "Tabe"=w309, "Connncet State"=w316) -> ("error out"=w313:errorcluster, "state"=w312:bool, "Connncet State out"=w311:T6)  [unwired: 3 in, 1 out]
        n102 = case shown="真" w312 {
          tunnel: w313 -> [w327 w338]
          tunnel: w311 -> [w326 w337]
          tunnel: w310 -> [_ w336]
          tunnel: w309 -> [w324 w333]
          tunnel: w308 -> [_ w332]
          tunnel: [w322 w329] -> w306
          tunnel: w307 -> [w325 _]
          tunnel: [w321 w328] -> w305
          frame False {
            n103 = call "DB insert array data（Feedback).vi"("Data"=w325, "error in (no error)"=w327, "index"=0, "table"=w324, "Connncet State"=w326) -> ("error out"=w322:errorcluster, "state"=w321:bool)  [unwired: 4 in, 1 out]
          }
          frame True {
            n104 = Bundle("date/time string"=w336) -> (w334:cluster{"date/time string":string})  [unwired: 1 in]
            n105 = To Variant(anything=w334) -> (Variant=w335:variant)
            n106 = call "DB Update Data(Feedback).vi"("Pos"=cluster{"index":i32, "Len":i32} {"index"=2, "Len"=1}, "Sel index"=0, "data"=w335, "error in (no error)"=w338, "Code"=w332, "table"=w333, "Connncet State"=w337) -> ("error out"=w329:errorcluster, "State"=w328:bool)  [unwired: 2 in, 1 out]
          }
        }
        n107 = call "Error cyc Times.vi"("error in (no error)"=w306, "Status in"=w305) -> ("error out"=w304:errorcluster, "Numeric"=w301:i32, "Cys Status"=w302:bool)  [unwired: 6 in, 1 out]
        n108 = Equal?(x=w301, y=2) -> (x = y?=w299:bool)
        n109 = Bundle By Name(cluster=w295, "information.cause"="更新服务器心跳失败！") -> (w294:T14)
        n110 = Select(t=string[] ["Heartbeat:Save Data", "Display Tip"], s=w299, f=string[] ["Heartbeat:Save Data"]) -> (s? t:f=w298:string[])
        n111 = Not(x=w302) -> (.not. x?=w303:bool)
      }
      frame "BR:Read Exc Signal" {
        n112 = Unbundle By Name(w348) -> ("Exc flag.Exchange Enable"=w350:bool)
        n113 = call-poly "Read Single Data.vi"("error in (no error)"=w354, "Tags"="Exchange_Model") -> ("error out"=w353:errorcluster, "Boolean"=w340:bool)  [unwired: 7 in, 1 out]
        n114 = call "Ture to Flase.vi"("in"=w340) -> ("Out"=w339:bool)  [unwired: 4 in]
        n115 = call <vilib>:"Boolean Crossing PtByPt.vi"("direction"=enum16{"either", "false-true", "true-false"}."false-true", "input"=w339) -> ("crossing"=w341:bool)  [unwired: 1 in]
        n116 = Select(t=TRUE, s=w350, f=w341) -> (s? t:f=w343:bool)
        n117 = Bundle By Name(cluster=w348, "Exc flag.Exchange Enable"=w343) -> (w347:T14)
        n118 = Select(t=string[] ["Exchange:Steps"], s=w343, f=string[] ["Exchange:Init Steps"]) -> (s? t:f=w342:string[])
      }
      frame "Exchange:Steps" {
      }
      frame "Exchange:Init Steps" {
        n119 = Unbundle By Name(w367) -> ("Exc flag.Exchange Enable"=w366:bool)
        n120 = call <vilib>:"Boolean Crossing PtByPt.vi"("direction"=enum16{"either", "false-true", "true-false"}."false-true", "input"=w366) -> ("crossing"=w363:bool)  [unwired: 1 in]
      }
      frame "Exchange:Ready ok" {
        n121 = Unbundle By Name(w370) -> ("Main.Local DB.Database.conn ref"=w376:T8)
        n122 = call <vilib>:"DB Tools Delete Data.vi"("condition"="", "error in (no error)"=w377, "table"="Exchange_Table", "connection reference"=w376) -> ("error out"=w375:errorcluster)  [unwired: 6 in, 1 out]
        n123 = Bundle By Name(cluster=w370, "ExcPN"=T9 {"Next PN"={"SN"="", "Model"="", "Pos"=0}, "PrePN"={"SN"="", "Model"="", "Pos"=0}}, "Exc flag.ms"=0.0) -> (w369:T14)
      }
      frame "Exchange:Reset Exc Signal" {
        # "TOP (1000)"
        n124 = Unbundle By Name(w401) -> ("Main.Local DB.Database.conn ref"=w402:T8, "Exc flag.Exchange Enable"=w380:bool)
        n125 = Not(x=w380) -> (.not. x?=w397:bool)
        n126 = call-poly "Write Single Data.vi"("error in (no error)"=w404, "Data"=w397, "Tags"="Exchange_Model") -> ("error out"=w396:errorcluster)  [unwired: 6 in, 2 out]
        n127 = call "Select top data.vi"("condition"="order by OnTime desc", "error in (no error)"=w396, "Row"=5, "table"="Online_Table", "connection reference"=w402) -> ("error out"=w392:errorcluster, "recordset data"=w391:variant[][])  [unwired: 4 in, 1 out]
        n128 = xnode "Database Variant To Data"("database variant"=w391, "error in (no error)"=w392, "type"=string[][] []) -> ("data"=w389:string[][], "error out"=w386:errorcluster)
        n129 = call "2D Table get 1D Rows.vi"("data"=w389) -> ("Rows"=w388:string[])  [unwired: 4 in]
        n130 = Index Array(array=w388, index #1=0 ("index"), index #2=3 ("索引")) -> (element #1=w384:string, element #2=w383:string)
        n131 = call <vilib>:"High Resolution Relative Seconds.vi"() -> ("relative seconds"=w381:dbl)
        n132 = Format Into String(format string="换型前SN:%1$s-Model:%2$s", error in=w386, w384, w383) -> (resulting string=w382:string, error out=w399:errorcluster)  [unwired: 1 in]
        n133 = Bundle By Name(cluster=w401, "Exc flag.ms"=w381, "ExcPN.PrePN.SN"=w384, "ExcPN.PrePN.Model"=w383, "information.cause"=w382, "Pos"=cluster{"Pre Pos":i32, "Next Pos":i32} {"Pre Pos"=-1, "Next Pos"=-1}) -> (w400:T14)
      }
      frame "Exchange:Get Next SN" {
        n134 = Unbundle By Name(w455) -> ("Main.Local DB.Database"=w449:T6, "ExcPN.PrePN.SN"=w452:string, "ExcPN.PrePN.Model"=w453:string, "ExcPN.Next PN.SN"=w451:string)
        n135 = Empty String/Path?(string/path=w451) -> (empty?=w450:bool)
        n136 = case shown="真" w450 {
          tunnel: w457 -> [w460 w489]
          tunnel: [w460 w475] -> w456
          tunnel: w455 -> [w459 w488]
          tunnel: [w459 w487] -> w454
          tunnel: w453 -> [_ w469]
          tunnel: w452 -> [_ w470]
          tunnel: w449 -> [_ w485]
          frame False {
          }
          frame True {
            w471 = ""
            w476 = 0 ("index")
            n137 = for {
              tunnel: string[] ["SN[1]", "Model[0]"] -> [w851] mode=indexing
              tunnel: w489 -> [w850]
              tunnel: [w849] -> w486
              tunnel: [w848] -> w483 mode=indexing
              tunnel: bool[] [TRUE, FALSE] -> [w847] mode=indexing
              n138 = call-poly "Read Single Data.vi"("error in (no error)"=w850, "Char/Str"=w847, "Tags"=w851) -> ("error out"=w849:errorcluster, "Data Byte"=w848:string)  [unwired: 6 in, 1 out]
            }
            n139 = Index Array(array=w483, index=0) -> (element=w482:string)
            n140 = call "DB select data(index).vi"("index"=w476, "Condtion"="order by OnTime desc", "error in (no error)"=w486, "Code"=w482, "Tabe"="Online_Table", "Connncet State"=w485) -> ("error out"=w479:errorcluster, "state"=w478:bool, "data"=w477:variant[][])  [unwired: 2 in, 1 out]
            n141 = case shown="真" w478 {
              tunnel: w479 -> [w491 w501]
              tunnel: w477 -> [_ w500]
              tunnel: w476 -> [_ w499]
              tunnel: [_ w495] -> w472
              tunnel: [_ w494] -> w473
              tunnel: [_ w493] -> w474
              tunnel: [w491 w492] -> w475
              frame False {
              }
              frame True {
                n142 = Index Array(array=w500, index (row)=w499) -> (element=w498:variant[])  [unwired: 1 in]
                n143 = xnode "Database Variant To Data"("database variant"=w498, "error in (no error)"=w501, "type"=T15 {"SN"="", "Frame"="", "Station"="", "Model"="", "Color"="", "OnTime"=timestamp(0 s since 1904-01-01), "OutTime"=timestamp(0 s since 1904-01-01), "Repaired"=0, "OnRepair"=FALSE, "Pstate"=""} ("Online_Table")) -> ("data"=w496:T15, "error out"=w492:errorcluster)
                n144 = Unbundle By Name(w496) -> ("SN"=w494:string, "Frame"=w493:string, "Model"=w495:string)
              }
            }
            n145 = Empty String/Path?(string/path=w474) -> (empty?=w468:bool)
            n146 = Select(t=w471, s=w468, f=w473) -> (s? t:f=w462:string)
            n147 = Select(t=w471, s=w468, f=w472) -> (s? t:f=w463:string)
            n148 = Not(x=w468) -> (.not. x?=w465:bool)
            n149 = Not Equal?(x=w470, y=w462) -> (x != y?=w467:bool)
            n150 = Not Equal?(x=w469, y=w463) -> (x != y?=w466:bool)
            n151 = Compound Arithmetic op=AND(w467, w466, w465) -> (w464:bool)
            n152 = case shown="真" w464 {
              tunnel: w488 -> [w842 w846]
              tunnel: [w842 w845] -> w487
              tunnel: w463 -> [_ w844]
              tunnel: w462 -> [_ w843]
              frame False {
              }
              frame True {
                n153 = Bundle By Name(cluster=w846, "ExcPN.Next PN.SN"=w843, "ExcPN.Next PN.Model"=w844) -> (w845:T14)
              }
            }
          }
        }
      }
      frame "Exchange:Serch SN Pos" {
        n154 = Unbundle By Name(w853) -> ("ExcPN.PrePN.SN"=w855:string, "ExcPN.Next PN.SN"=w854:string)
        n155 = Empty String/Path?(string/path=w855) -> (empty?=w857:bool)
        n156 = Empty String/Path?(string/path=w854) -> (empty?=w858:bool)
        n157 = And(x=w857, y=w858) -> (x .and. y?=w856:bool)
        n158 = case shown="假" w856 {
          tunnel: w860 -> [w875 w890]
          tunnel: [w873 w890] -> w859
          tunnel: w855 -> [w872 _]
          tunnel: w854 -> [w871 _]
          tunnel: w853 -> [w868 w888]
          tunnel: [w867 w889] -> w852
          frame False {
            n159 = Build Array(w872, w871) -> (w869:string[])
            n160 = for {
              tunnel: w875 -> [w886]
              tunnel: string[] ["SN[0]", "SN[1]", "SN[2]", "SN[3]", "SN[4]", "SN[5]", "SN[6]", "SN[7]", "SN[8]", "SN[9]", "SN[10]", "SN[11]", "SN[12]"] -> [w885] mode=indexing
              tunnel: [w884] -> w873
              tunnel: [w883] -> w870 mode=indexing
              tunnel: TRUE -> [w882]
              n161 = call-poly "Read Single Data.vi"("error in (no error)"=w886, "Char/Str"=w882, "Tags"=w885) -> ("error out"=w884:errorcluster, "Data Byte"=w883:string)  [unwired: 6 in, 1 out]
            }
            n162 = for {
              tunnel: w870 -> [w881]
              tunnel: w869 -> [w880] mode=indexing
              tunnel: [w876] -> w866 mode=indexing
              n163 = Search 1D Array(1D array=w881, element=w880) -> (index of element=w878:i32)  [unwired: 1 in]
              n164 = Empty String/Path?(string/path=w880) -> (empty?=w879:bool)
              n165 = Select(t=-1, s=w879, f=w878) -> (s? t:f=w876:i32)
            }
            n166 = Index Array(array=w866, index #1=0 ("index")) -> (element #1=w864:i32, element #2=w863:i32)  [unwired: 1 in]
            n167 = Bundle By Name(cluster=w868, "ExcPN.PrePN.Pos"=w864, "ExcPN.Next PN.Pos"=w863) -> (w867:T14)
          }
          frame True {
            w887 = -1
            n168 = Bundle By Name(cluster=w888, "ExcPN.Next PN.Pos"=w887, "ExcPN.PrePN.Pos"=w887) -> (w889:T14)
          }
        }
      }
      frame "Exchange:Exc PrePN Table" {
        # "%1$s"
        n169 = Unbundle By Name(w903) -> ("ExcPN.PrePN.SN"=w897:string, "Exchange Table"=w914:T10, "ExcPN.PrePN.Model"=w915:string, "Main.FTT TV"=w916:string, "ExcPN.PrePN.Pos"=w891:i32, "Main.Local DB.Database"=w917:T6, "Pos.Pre Pos"=w895:i32)
        n170 = Greater Or Equal To 0?(x=w891) -> (x >= 0?=w893:bool)
        n171 = Not Equal?(x=w891, y=w895) -> (x != y?=w892:bool)
        n172 = And(x=w892, y=w893) -> (x .and. y?=w894:bool)
        n173 = case shown="真" w894 {
          tunnel: w919 -> [w922 w941]
          tunnel: "Station[%1$d]" -> [w923 w940]
          tunnel: w917 -> [_ w936]
          tunnel: w916 -> [_ w931]
          tunnel: w915 -> [_ w930]
          tunnel: w914 -> [_ w928]
          tunnel: [w922 w927] -> w913
          tunnel: [TRUE w926] -> w912
          tunnel: [w923 w925] -> w898
          tunnel: w891 -> [_ w924]
          frame False {
          }
          frame True {
            w929 = "Exchange_Table"
            n174 = Format Into String(format string=w940, error in=w941, w924) -> (resulting string=w938:string, error out=w939:errorcluster)  [unwired: 1 in]
            n175 = call-poly "Read Single Data.vi"("error in (no error)"=w939, "Tags"=w938) -> ("error out"=w937:errorcluster, "Data Byte"=w925:string)  [unwired: 7 in, 1 out]
            n176 = call "DB select data(index).vi"("index"=2, "error in (no error)"=w937, "Code"=w925, "Tabe"=w929, "Connncet State"=w936) -> ("error out"=w935:errorcluster, "state"=w933:bool, "Connncet State out"=w932:T6)  [unwired: 3 in, 1 out]
            n177 = case shown="假" w933 {
              tunnel: w935 -> [w950 w956]
              tunnel: w932 -> [w949 _]
              tunnel: w931 -> [w954 _]
              tunnel: w925 -> [w953 _]
              tunnel: w930 -> [w952 _]
              tunnel: w929 -> [w948 _]
              tunnel: w928 -> [w946 _]
              tunnel: [w943 w956] -> w927
              tunnel: [w942 TRUE] -> w926
              frame False {
                n178 = Get Date/Time In Seconds() -> (seconds since 1Jan1904=w951:timestamp)
                n179 = Bundle By Name(cluster=w946, "LineName"=w954, "Model"=w952, "Station"=w953, "StartTime"=w951) -> (w945:T10)
                n180 = call "Exchange Table array.vi"("Exchange Table"=w945) -> ("appended array"=w944:string[])  [unwired: 4 in]
                n181 = call "DB insert array data（Feedback).vi"("Data"=w944, "error in (no error)"=w950, "index"=3, "table"=w948, "Connncet State"=w949) -> ("error out"=w943:errorcluster, "state"=w942:bool)  [unwired: 4 in, 1 out]
              }
              frame True {
              }
            }
          }
        }
        n182 = call "Error cyc Times.vi"("error in (no error)"=w913, "Status in"=w912) -> ("error out"=w901:errorcluster, "Numeric"=w909:i32, "Cys Status"=w911:bool)  [unwired: 6 in, 1 out]
        n183 = Equal?(x=w909, y=2) -> (x = y?=w907:bool)
        n184 = Format Into String(format string="产品换型%1$s-SN:%2$s数据存储异常！", error in=w901, w898, w897) -> (resulting string=w896:string, error out=w900:errorcluster)  [unwired: 1 in]
        n185 = Bundle By Name(cluster=w903, "information.cause"=w896, "Pos.Pre Pos"=w891) -> (w902:T14)
        n186 = Not(x=w911) -> (.not. x?=w910:bool)
        n187 = Select(t=string[] ["Exchange:Exc PrePN Table", "Display Tip"], s=w907, f=string[] ["Exchange:Exc PrePN Table"]) -> (s? t:f=w906:string[])
      }
      frame "Exchange:Exc NextPN Table Update" {
        n188 = Unbundle By Name(w959) -> ("ExcPN.Next PN.SN"=w966:string, "Exchange Table"=w980:T10, "ExcPN.Next PN.Pos"=w957:i32, "Main.Local DB.Database"=w982:T6, "Pos.Next Pos"=w963:i32)
        n189 = Not Equal?(x=w963, y=w957) -> (x != y?=w961:bool)
        n190 = Greater Or Equal To 0?(x=w957) -> (x >= 0?=w960:bool)
        n191 = And(x=w961, y=w960) -> (x .and. y?=w962:bool)
        n192 = case shown="真" w962 {
          tunnel: w983 -> [w986 w999]
          tunnel: w982 -> [_ w991]
          tunnel: w957 -> [_ w998]
          tunnel: "Station[%1$d]" -> [w984 w997]
          tunnel: w980 -> [_ w992]
          tunnel: [w986 w989] -> w978
          tunnel: [TRUE ("State") w988] -> w977
          tunnel: [w984 w987] -> w967
          frame False {
          }
          frame True {
            w990 = "Exchange_Table"
            n193 = Format Into String(format string=w997, error in=w999, w998) -> (resulting string=w1002:string, error out=w1003:errorcluster)  [unwired: 1 in]
            n194 = call-poly "Read Single Data.vi"("error in (no error)"=w1003, "Tags"=w1002) -> ("error out"=w1001:errorcluster, "Data Byte"=w987:string)  [unwired: 7 in, 1 out]
            n195 = call "DB select data(index).vi"("index"=2, "Condtion"="order by StartTime", "error in (no error)"=w1001, "Code"=w987, "Tabe"=w990, "Connncet State"=w991) -> ("error out"=w994:errorcluster, "state"=w993:bool, "data"=w995:variant[][])  [unwired: 2 in, 1 out]
            n196 = case shown="真" w993 {
              tunnel: w995 -> [_ w1024]
              tunnel: w994 -> [w1005 w1022]
              tunnel: w992 -> [_ w1020]
              tunnel: w991 -> [_ w1016]
              tunnel: w990 -> [_ w1015]
              tunnel: [w1005 w1007] -> w989
              tunnel: [TRUE ("State") w1006] -> w988
              frame False {
              }
              frame True {
                n197 = Index Array(array=w1024, index (row)=0) -> (element=w1021:variant[])  [unwired: 1 in]
                n198 = xnode "Database Variant To Data"("database variant"=w1021, "error in (no error)"=w1022, "type"=w1020) -> ("data"=w1019:T10, "error out"=w1017:errorcluster)
                n199 = Get Date/Time In Seconds() -> (seconds since 1Jan1904=w1013:timestamp)
                n200 = Unbundle By Name(w1019) -> ("Station"=w1014:string, "StartTime"=w1018:timestamp)
                n201 = Subtract(x=w1013, y=w1018) -> (x-y=w1012:dbl)
                n202 = Bundle("seconds since 1Jan1904"=w1013, w1012) -> (w1011:cluster{"seconds since 1Jan1904":timestamp, dbl})  [unwired: 1 in]
                n203 = To Variant(anything=w1011) -> (Variant=w1010:variant)
                n204 = call "DB Update Data(Feedback).vi"("Pos"=cluster{"index":i32, "Len":i32} {"index"=4, "Len"=2}, "Sel index"=2, "data"=w1010, "error in (no error)"=w1017, "Code"=w1014, "table"=w1015, "Connncet State"=w1016) -> ("error out"=w1007:errorcluster, "State"=w1006:bool)  [unwired: 2 in, 1 out]
              }
            }
          }
        }
        n205 = call "Error cyc Times.vi"("error in (no error)"=w978, "Status in"=w977) -> ("error out"=w970:errorcluster, "Numeric"=w976:i32, "Cys Status"=w964:bool)  [unwired: 6 in, 1 out]
        n206 = Bundle By Name(cluster=w959, "Pos.Next Pos"=w957) -> (w958:T14)
        n207 = Equal?(x=w976, y=2) -> (x = y?=w974:bool)
        n208 = Format Into String(format string="产品换型%1$s-SN:%2$s数据存储异常！", error in=w970, w967, w966) -> (error out=w969:errorcluster)  [unwired: 1 in, 1 out]
        n209 = Select(t=string[] ["Exchange:Exc NextPN Table Update", "Display Tip"], s=w974, f=string[] ["Exchange:Exc NextPN Table Update"]) -> (s? t:f=w972:string[])
        n210 = Not(x=w964) -> (.not. x?=w965:bool)
      }
      frame "Exchange:End Judge" {
        n211 = Unbundle By Name(w1243) -> ("Main.ExchangeTime"=w1241:i32, "Exc flag.Exchange Enable"=w1245:bool, "Exc flag.ms"=w1260:dbl, "ExcPN.PrePN.SN"=w1257:string, "ExcPN.Next PN.SN"=w1256:string, "Main.Local DB.Database"=w1253:T6)
        n212 = call <vilib>:"High Resolution Relative Seconds.vi"() -> ("relative seconds"=w1259:dbl)
        n213 = Build Array(w1257, w1256) -> (w1252:string[])
        n214 = for {
          tunnel: w1254 -> [w1267]
          tunnel: w1253 -> [w1266]
          tunnel: w1252 -> [w1264] mode=indexing
          tunnel: "Online_Table" -> [w1263]
          tunnel: [w1262] -> w1249 mode=indexing
          tunnel: [w1261] -> w1250
          n215 = Empty String/Path?(string/path=w1264) -> (empty?=w1265:bool)
          n216 = case shown="假" w1265 {
            tunnel: w1267 -> [w1275 w1276]
            tunnel: w1266 -> [w1274 _]
            tunnel: w1264 -> [w1273 _]
            tunnel: w1263 -> [w1272 _]
            tunnel: [w1269 _] -> w1262
            tunnel: [w1268 w1276] -> w1261
            frame False {
              n217 = call "DB select data(index).vi"("index"=0, "Condtion"="and Pstate<>''", "error in (no error)"=w1275, "Code"=w1273, "Tabe"=w1272, "Connncet State"=w1274) -> ("error out"=w1268:errorcluster, "state"=w1269:bool)  [unwired: 2 in, 2 out]
            }
            frame True {
            }
          }
        }
        n218 = Subtract(x=w1259, y=w1260) -> (x-y=w1258:dbl)
        n219 = Greater?(x=w1258, y=w1241) -> (0:w1248:bool)
        n220 = And Array Elements(Boolean array=w1249) -> (logical AND=w1242:bool)
        n221 = Or(x=w1248, y=w1242) -> (x .or. y?=w1246:bool)
        n222 = And(x=w1245, y=w1246) -> (x .and. y?=w1244:bool)
      }
      frame "Exchange:Read OutTime" {
        n223 = Unbundle By Name(w1286) -> ("Main.FTT TV"=w1280:string, "Main.EOL Path"=w1284:path, "Main.Local DB.Database"=w1296:T6, "ExcPN.Next PN.Model"=w1279:string, "ExcPN.PrePN.Model"=w1278:string)
        n224 = call "Get  PreCurrentTime.vi"("hour"=2, "error in (no error)"=w1305) -> ("CurrStr"=w1303:string, "PreStr"=w1302:string, "error out"=w1306:errorcluster)  [unwired: 9 in, 2 out]
        n225 = call "Build exc Msg.vi"("error in (no error)"=w1306, "PreT"=w1302, "CurrT"=w1303) -> ("error out"=w1299:errorcluster, "PreMode"=w1300:string, "CurrMode"=w1301:string)  [unwired: 6 in]
        n226 = Build Array(w1279, w1278) -> (w1283:string[])
        n227 = Build Array(w1301, w1300) -> (w1297:string[])
        n228 = for {
          tunnel: w1299 -> [w1687]
          tunnel: "Online_Table" -> [w1685]
          tunnel: w1297 -> [w1684] mode=indexing
          tunnel: w1283 -> [w1683]
          tunnel: w1296 -> [w1680]
          tunnel: [w1679] -> w1295 mode=indexing
          tunnel: [w1678] -> w1289
          tunnel: [w1675] -> w1290 mode=indexing
          i -> [w1681]
          n229 = Index Array(array=w1683, index=w1681) -> (element=w1682:string)
          n230 = call "DB select data(index).vi"("index"=3, "Condtion"=w1684, "error in (no error)"=w1687, "Code"=w1682, "Tabe"=w1685, "Connncet State"=w1680) -> ("error out"=w1678:errorcluster, "state"=w1679:bool, "data"=w1677:variant[][])  [unwired: 2 in, 1 out]
          n231 = Index Array(array=w1677, index (row)=0) -> (element=w1675:variant[])  [unwired: 1 in]
        }
        n232 = Empty Array?(array=w1295) -> (empty?=w1294:bool)
        n233 = Not(x=w1294) -> (.not. x?=w1292:bool)
        n234 = And Array Elements(Boolean array=w1295) -> (logical AND=w1293:bool)
        n235 = And(x=w1292, y=w1293) -> (x .and. y?=w1291:bool)
        n236 = case shown="假" w1291 {
          tunnel: w1290 -> [_ w1327]
          tunnel: w1289 -> [w1316 w1328]
          tunnel: [w1312 w1324] -> w1287
          tunnel: [w1315 w1323] -> w1288
          tunnel: w1284 -> [w1313 _]
          tunnel: w1283 -> [w1314 _]
          tunnel: [w1308 w1318] -> w1282
          tunnel: [w1307 w1317] -> w1281
          frame False {
            n237 = call "Eol Exc Time.vi"("error in (no error)"=w1316, "Mode"=w1314, "base"=w1313) -> ("error out"=w1315:errorcluster, "Array"=w1311:timestamp[], "Numeric"=w1312:dbl)  [unwired: 6 in]
            n238 = Index Array(array=w1311, index #1=1 ("index"), index #2=0 ("index")) -> (element #1=w1308:timestamp, element #2=w1307:timestamp)
          }
          frame True {
            n239 = xnode "Database Variant To Data"("database variant"=w1327, "error in (no error)"=w1328, "type"=T15[] []) -> ("data"=w1321:T15[], "error out"=w1323:errorcluster)
            n240 = Index Array(array=w1321, index #1=0, index #2=1) -> (element #1=w1320:T15, element #2=w1319:T15)
            n241 = Unbundle By Name(w1320) -> ("OutTime"=w1318:timestamp)
            n242 = Unbundle By Name(w1319) -> ("OutTime"=w1317:timestamp)
            n243 = Subtract(x=w1318, y=w1317) -> (x-y=w1324:dbl)
          }
        }
        n244 = Bundle By Name(cluster=w1286, "BR.NextPN"=w1279, "BR.PrePN"=w1278, "BR.Line Name"=w1280, "BR.End Time"=w1282, "excT"=w1287, "BR.Start Tine"=w1281) -> (w1285:T14)
      }
      frame "Exchange:Get Esc SubTimeMax" {
        n245 = Unbundle By Name(w1701) -> ("excT"=w1688:dbl, "BR"=w1705:T13, "Main.FTT TV"=w1704:string, "Main.Local DB.Database"=w1697:T6, "Exchange Table"=w1707:T10, "ExcPN"=w1703:T9, "ExcPN.PrePN.Model"=w1695:string, "ExcPN.Next PN.Model"=w1693:string)
        n246 = call "DB select data(index).vi"("index"=1, "error in (no error)"=w1712, "Code"=w1695, "Tabe"="Exchange_Table", "Connncet State"=w1697) -> ("error out"=w1710:errorcluster, "data"=w1709:variant[][])  [unwired: 3 in, 2 out]
        n247 = Empty Array?(array=w1709) -> (empty?=w1708:bool)
        n248 = case shown="假" w1708 {
          tunnel: w1710 -> [w1726 w1984]
          tunnel: w1709 -> [w1725 _]
          tunnel: w1707 -> [w1724 _]
          tunnel: w1705 -> [w1721 w1981]
          tunnel: w1704 -> [_ _]
          tunnel: w1703 -> [_ _]
          tunnel: [w1720 w1984] -> w1702
          tunnel: [w1719 w1979] -> w1699
          tunnel: [w1713 w1972] -> w1689
          tunnel: w1688 -> [w1715 w1978]
          frame False {
            n249 = Build Array(w1724) -> (w1723:T10[])
            n250 = xnode "Database Variant To Data"("database variant"=w1725, "error in (no error)"=w1726, "type"=w1723) -> ("data"=w1722:T10[], "error out"=w1720:errorcluster)
            n251 = for {
              tunnel: w1722 -> [w1749] mode=indexing
              tunnel: [w1748] -> w1718 mode=indexing
              n252 = Unbundle By Name(w1749) -> ("SubTime"=w1748:dbl)
            }
            n253 = call "Exc time Result.vi"("SubVI"=w1718) -> ("Pos"=w1717:i32, "Tip"=w1714:string, "Status"=w1716:bool)  [unwired: 8 in]
            n254 = case shown="假" w1716 {
              tunnel: w1717 -> [w1735 _]
              tunnel: w1722 -> [w1734 _]
              tunnel: w1721 -> [w1733 w1747]
              tunnel: [w1728 w1746] -> w1719
              tunnel: w1715 -> [_ w1742]
              tunnel: w1714 -> [w1727 _]
              tunnel: [w1727 w1736] -> w1713
              frame False {
                n255 = Index Array(array=w1734, index=w1735) -> (element=w1732:T10)
                n256 = Unbundle By Name(w1732) -> ("StartTime"=w1731:timestamp, "EndTime"=w1730:timestamp)
                n257 = Bundle By Name(cluster=w1733, "Start Tine"=w1731, "End Time"=w1730, "Status"=TRUE) -> (w1728:T13)
              }
              frame True {
                n258 = Divide(x=w1742, y=60.0) -> (x/y=w1740:dbl)
                n259 = In Range and Coerce(upper limit=1800.0, x=w1742, lower limit=480.0) -> (In Range?=w1743:bool)  [unwired: 1 out]
                n260 = Number To Decimal String(number=w1740) -> (decimal integer string=w1737:string)  [unwired: 1 in]
                n261 = Bundle By Name(cluster=w1747, "Status"=w1743) -> (w1746:T13)
                n262 = Concatenate Strings("换型时间", w1737, "min" ("string")) -> (w1736:string)
              }
            }
          }
          frame True {
            n263 = In Range and Coerce(upper limit=1800.0, x=w1978, lower limit=480.0) -> (In Range?=w1980:bool)  [unwired: 1 out]
            n264 = Divide(x=w1978, y=60.0) -> (x/y=w1976:dbl)
            n265 = Number To Decimal String(number=w1976) -> (decimal integer string=w1974:string)  [unwired: 1 in]
            n266 = Concatenate Strings("换型时间", w1974, "min" ("string")) -> (w1972:string)
            n267 = Bundle By Name(cluster=w1981, "Status"=w1980) -> (w1979:T13)
          }
        }
        n268 = Concatenate Strings(w1693, w1689) -> (w1692:string)
        n269 = Unbundle By Name(w1699) -> ("Status"=w1698:bool)
        n270 = Bundle By Name(cluster=w1701, "Exc flag.ms"=0.0, "Exc flag.Exchange Enable"=FALSE, "BR"=w1699, "information.cause"=w1692) -> (w1700:T14)
      }
      frame "Exchange:Server_exc Table" {
        w2011 = "AJ_Exchange_Run"
        n271 = Unbundle By Name(w1997) -> ("ExcPN.Next PN.Model"=w1993:string, "BR"=w2010:T13, "Main.Remote DB.Database"=w2016:T6, "BR.Line Name"=w1986:string, "BR.PrePN"=w1985:string)
        n272 = call "DB select data(index).vi"("index"=0, "error in (no error)"=w2017, "Code"=w1986, "Tabe"=w2011, "Connncet State"=w2016) -> ("error out"=w2014:errorcluster, "state"=w2013:bool, "Connncet State out"=w2012:T6)  [unwired: 3 in, 1 out]
        n273 = case shown="真" w2013 {
          tunnel: w2014 -> [w2025 w2052]
          tunnel: w2012 -> [w2024 w2051]
          tunnel: w2011 -> [w2027 w2049]
          tunnel: w2010 -> [w2022 w2041]
          tunnel: w1986 -> [_ w2046]
          tunnel: "AJ_Exchange_History" -> [w2026 w2042]
          tunnel: [w2020 w2040] -> w2008
          tunnel: [w2018 w2039] -> w2007
          tunnel: w1985 -> [_ w2036]
          frame False {
            n274 = call "Server Exc_table.vi"("BR"=w2022) -> ("appended array"=w2021:string[])  [unwired: 10 in]
            n275 = Build Array(w2027, w2026) -> (w2023:string[])
            n276 = for {
              tunnel: w2025 -> [w2034]
              tunnel: w2024 -> [w2033]
              tunnel: w2023 -> [w2032] mode=indexing
              tunnel: w2021 -> [w2030]
              tunnel: [w2029] -> w2020
              tunnel: [w2028] -> w2019 mode=indexing
              n277 = call "DB insert array data（Feedback).vi"("Data"=w2030, "error in (no error)"=w2034, "index"=3, "table"=w2032, "Connncet State"=w2033) -> ("error out"=w2029:errorcluster, "state"=w2028:bool)  [unwired: 4 in, 1 out]
            }
            n278 = And Array Elements(Boolean array=w2019) -> (logical AND=w2018:bool)
          }
          frame True {
            n279 = To Variant(anything=w2041) -> (Variant=w2050:variant)
            n280 = Concatenate Strings("and PrePN='" ("Sel"), w2036, "'" ("string")) -> (w2037:string)
            n281 = call "DB Update Data(Feedback_nc).vi"("Connncet State"=w2051, "data"=w2050, "Sel"=w2037, "table"=w2049, "Code"=w2046, "error in (no error)"=w2052, "Sel index"=0, "Pos"=cluster{"index":i32, "Len":i32} {"index"=0, "Len"=6}) -> ("Connncet State out"=w2043:T6, "State"=w2044:bool, "error out"=w2045:errorcluster)  [unwired: 5 in]
            n282 = case shown="真" w2044 {
              tunnel: w2045 -> [w2054 w2062]
              tunnel: w2043 -> [_ w2061]
              tunnel: w2042 -> [_ w2060]
              tunnel: w2041 -> [_ w2058]
              tunnel: [w2054 w2056] -> w2040
              tunnel: [FALSE w2055] -> w2039
              frame False {
              }
              frame True {
                n283 = call "Server Exc_table.vi"("BR"=w2058) -> ("appended array"=w2057:string[])  [unwired: 10 in]
                n284 = call "DB insert array data（Feedback).vi"("Data"=w2057, "error in (no error)"=w2062, "index"=3, "table"=w2060, "Connncet State"=w2061) -> ("error out"=w2056:errorcluster, "state"=w2055:bool)  [unwired: 4 in, 1 out]
              }
            }
          }
        }
        n285 = call "Error cyc Times.vi"("error in (no error)"=w2008, "Status in"=w2007) -> ("error out"=w1995:errorcluster, "Numeric"=w2003:i32, "Cys Status"=w2004:bool, "Status out"=w1990:bool)  [unwired: 6 in]
        n286 = Select(t="%1$s换型完成！", s=w1990, f="%1$s换型服务器更新数据失败！") -> (s? t:f=w1988:string)
        n287 = Equal?(x=w2003, y=2) -> (x = y?=w2001:bool)
        n288 = Format Into String(format string=w1988, error in=w1995, w1993) -> (resulting string=w1992:string, error out=w1994:errorcluster)  [unwired: 1 in]
        n289 = Not(x=w1990) -> (.not. x?=w1991:bool)
        n290 = Bundle By Name(cluster=w1997, "information.cause"=w1992, "information.Status"=w1991) -> (w1996:T14)
        n291 = Select(t=string[] ["Exchange:Server_exc Table", "Display Tip"], s=w2001, f=string[] ["Exchange:Server_exc Table"]) -> (s? t:f=w2000:string[])
        n292 = Not(x=w2004) -> (.not. x?=w2005:bool)
      }
      frame "BR:Steps" {
      }
      frame "BR:Read Server BR" {
        n293 = Unbundle By Name(w2072) -> ("Main.Remote DB.Database"=w2078:T6, "Main.FTT TV"=w2076:string)
        n294 = call "DB select data(index).vi"("index"=0, "error in (no error)"=w2079, "Code"=w2076, "Tabe"="AJ_RunV", "Connncet State"=w2078) -> ("error out"=w2073:errorcluster, "state"=w2068:bool, "data"=w2074:variant[][])  [unwired: 3 in, 1 out]
        n295 = case shown="假" w2068 {
          tunnel: w2074 -> [_ w2103]
          tunnel: w2073 -> [w2081 w2101]
          tunnel: w2072 -> [w2080 w2097]
          tunnel: [w2080 w2096] -> w2071
          tunnel: [w2081 w2090] -> w2070
          frame False {
          }
          frame True {
            n296 = Index Array(array=w2103, index (row)=0) -> (element=w2100:variant[])  [unwired: 1 in]
            n297 = xnode "Database Variant To Data"("database variant"=w2100, "error in (no error)"=w2101, "type"=T11 {"LineName"="", "ProjectName"="", "AcutalOuput"=0, "ProStatus"="", "PlanOutput"=0, "ProTime"=0, "ShiftFlag"=""} ("AJ Run")) -> ("data"=w2089:T11, "error out"=w2098:errorcluster)
            n298 = Unbundle By Name(w2089) -> ("ProStatus"=w2094:string, "PlanOutput"=w2093:u32, "ShiftFlag"=w2083:string)
            n299 = call "Global FTT Data.vi"("error in (no error)"=w2098, "Mode"=enum16{"Read", "Write"}."Read") -> ("error out"=w2085:errorcluster, "Cluster"=w2088:T18)  [unwired: 8 in]
            n300 = call "Class Flag to Eum.vi"("error in (no error)"=w2085, "Str"=w2083) -> ("error out"=w2084:errorcluster, "Class"=w2082:enum16{"Big", "Small"})  [unwired: 8 in]
            n301 = Unbundle By Name(w2088) -> ("Display.Actual"=w2087:dbl, "Display.Model"=w2086:string)
            n302 = Bundle By Name(cluster=w2088, "Display.Line State"=w2094, "Display.Plan"=w2093, "Class"=w2082) -> (w2092:T18)
            n303 = Bundle By Name(cluster=w2097, "AJ Run.AcutalOuput"=w2087, "AJ Run.ProjectName"=w2086) -> (w2096:T14)
            n304 = call "Global FTT Data.vi"("error in (no error)"=w2084, "Mode"=enum16{"Read", "Write"}."Write", "Display"=w2092) -> ("error out"=w2090:errorcluster)  [unwired: 7 in, 1 out]
          }
        }
      }
      frame "BR:Update Server Data" {
        n305 = Unbundle By Name(w2325) -> ("AJ Run"=w2337:T11, "Main.Remote DB.Database"=w2342:T6, "Main.FTT TV"=w2340:string)
        n306 = First Call?() -> (First Call?: T/F=w2339:bool)
        n307 = case shown="真" w2339 {
          tunnel: w2343 -> [w2355 w2370]
          tunnel: w2342 -> [w2354 w2369]
          tunnel: "AJ_Run" -> [w2351 w2364]
          tunnel: w2340 -> [w2352 w2363]
          tunnel: w2337 -> [w2353 w2358]
          tunnel: [w2349 w2362] -> w2336
          tunnel: [w2348 w2361] -> w2335
          frame False {
            n308 = call "BR Update Data.vi"("AJ Run in"=w2353) -> ("AJ Run"=w2347:T11)  [unwired: 5 in, 1 out]
            n309 = Unbundle By Name(w2347) -> ("ProjectName"=w2345:string, "AcutalOuput"=w2346:u32)
            n310 = Bundle("ProjectName"=w2345, "AcutalOuput"=w2346) -> (w2344:cluster{"ProjectName":string, "AcutalOuput":u32})  [unwired: 1 in]
            n311 = To Variant(anything=w2344) -> (Variant=w2356:variant)
            n312 = call "DB Update Data(Feedback).vi"("Pos"=cluster{"index":i32, "Len":i32} {"index"=1, "Len"=2}, "Sel index"=0, "data"=w2356, "error in (no error)"=w2355, "Code"=w2352, "table"=w2351, "Connncet State"=w2354) -> ("error out"=w2349:errorcluster, "State"=w2348:bool)  [unwired: 2 in, 1 out]
          }
          frame True {
            n313 = call "BR Update Data.vi"("AJ Run in"=w2358) -> ("appended array"=w2359:string[], "AJ Run"=w2360:T11)  [unwired: 5 in]
            n314 = call "DB select data(index).vi"("index"=0, "error in (no error)"=w2370, "Code"=w2363, "Tabe"=w2364, "Connncet State"=w2369) -> ("error out"=w2367:errorcluster, "state"=w2366:bool, "Connncet State out"=w2365:T6)  [unwired: 3 in, 1 out]
            n315 = case shown="真" w2366 {
              tunnel: w2367 -> [w2377 w2390]
              tunnel: w2365 -> [w2376 w2389]
              tunnel: w2364 -> [w2375 w2388]
              tunnel: w2363 -> [_ w2387]
              tunnel: [w2372 w2384] -> w2362
              tunnel: [w2371 w2382] -> w2361
              tunnel: w2360 -> [_ w2381]
              tunnel: w2359 -> [w2373 _]
              frame False {
                n316 = call "DB insert array data（Feedback).vi"("Data"=w2373, "error in (no error)"=w2377, "index"=0, "table"=w2375, "Connncet State"=w2376) -> ("error out"=w2372:errorcluster, "state"=w2371:bool)  [unwired: 4 in, 1 out]
              }
              frame True {
                n317 = Unbundle By Name(w2381) -> ("ProjectName"=w2380:string, "AcutalOuput"=w2379:u32)
                n318 = Bundle("ProjectName"=w2380, "AcutalOuput"=w2379) -> (w2378:cluster{"ProjectName":string, "AcutalOuput":u32})  [unwired: 1 in]
                n319 = To Variant(anything=w2378) -> (Variant=w2383:variant)
                n320 = call "DB Update Data(Feedback).vi"("Pos"=cluster{"index":i32, "Len":i32} {"index"=1, "Len"=2}, "Sel index"=0, "data"=w2383, "error in (no error)"=w2390, "Code"=w2387, "table"=w2388, "Connncet State"=w2389) -> ("error out"=w2384:errorcluster, "State"=w2382:bool)  [unwired: 2 in, 1 out]
              }
            }
          }
        }
        n321 = call "Error cyc Times.vi"("error in (no error)"=w2336, "Status in"=w2335) -> ("error out"=w2334:errorcluster, "Numeric"=w2331:i32, "Cys Status"=w2332:bool)  [unwired: 6 in, 1 out]
        n322 = Equal?(x=w2331, y=2) -> (x = y?=w2329:bool)
        n323 = Select(t=string[] ["BR:Update Server Data", "Display Tip"], s=w2329, f=string[] ["BR:Update Server Data"]) -> (s? t:f=w2326:string[])
        n324 = Not(x=w2332) -> (.not. x?=w2333:bool)
      }
      frame "BR:Update AJ_EndRun" {
        n325 = call "Global Mes Triger.vi"("error in (no error)"=w2399, "R/S"=FALSE) -> ("error out"=w2397:errorcluster, "Var out"=w2396:T19)  [unwired: 8 in]
        n326 = Unbundle By Name(w2403) -> ("AJ Run"=w2393:T11, "Main.Remote DB.Database"=w2405:T6, "Main.FTT TV"=w2407:string)
        n327 = Unbundle By Name(w2396) -> ("Model"=w2391:string)
        n328 = Bundle By Name(cluster=w2393, "ProjectName"=w2391) -> (w2392:T11)
        n329 = Empty String/Path?(string/path=w2391) -> (empty?=w2395:bool)
        n330 = First Call?() -> (First Call?: T/F=w2408:bool)
        n331 = Select(t=w2393, s=w2395, f=w2392) -> (s? t:f=w2394:T11)
        n332 = case shown="真" w2408 {
          tunnel: w2397 -> [w2428 w2443]
          tunnel: w2405 -> [w2427 w2442]
          tunnel: "AJ_EndRun" -> [w2424 w2437]
          tunnel: w2407 -> [w2425 w2436]
          tunnel: w2394 -> [w2426 w2431]
          tunnel: [w2422 w2435] -> w2409
          tunnel: [w2421 w2434] -> w2410
          frame False {
            n333 = call "BR Update Data.vi"("AJ Run in"=w2426) -> ("AJ Run"=w2420:T11)  [unwired: 5 in, 1 out]
            n334 = Unbundle By Name(w2420) -> ("ProjectName"=w2418:string, "AcutalOuput"=w2419:u32)
            n335 = Bundle("ProjectName"=w2418, "AcutalOuput"=w2419) -> (w2417:cluster{"ProjectName":string, "AcutalOuput":u32})  [unwired: 1 in]
            n336 = To Variant(anything=w2417) -> (Variant=w2429:variant)
            n337 = call "DB Update Data(Feedback).vi"("Pos"=cluster{"index":i32, "Len":i32} {"index"=1, "Len"=2}, "Sel index"=0, "data"=w2429, "error in (no error)"=w2428, "Code"=w2425, "table"=w2424, "Connncet State"=w2427) -> ("error out"=w2422:errorcluster, "State"=w2421:bool)  [unwired: 2 in, 1 out]
          }
          frame True {
            n338 = call "BR Update Data.vi"("AJ Run in"=w2431) -> ("appended array"=w2432:string[], "AJ Run"=w2433:T11)  [unwired: 5 in]
            n339 = call "DB select data(index).vi"("index"=0, "error in (no error)"=w2443, "Code"=w2436, "Tabe"=w2437, "Connncet State"=w2442) -> ("error out"=w2440:errorcluster, "state"=w2439:bool, "Connncet State out"=w2438:T6)  [unwired: 3 in, 1 out]
            n340 = case shown="真" w2439 {
              tunnel: w2440 -> [w2450 w2463]
              tunnel: w2438 -> [w2449 w2462]
              tunnel: w2437 -> [w2448 w2461]
              tunnel: w2436 -> [_ w2460]
              tunnel: [w2445 w2457] -> w2435
              tunnel: [w2444 w2455] -> w2434
              tunnel: w2433 -> [_ w2454]
              tunnel: w2432 -> [w2446 _]
              frame False {
                n341 = call "DB insert array data（Feedback).vi"("Data"=w2446, "error in (no error)"=w2450, "index"=0, "table"=w2448, "Connncet State"=w2449) -> ("error out"=w2445:errorcluster, "state"=w2444:bool)  [unwired: 4 in, 1 out]
              }
              frame True {
                n342 = Unbundle By Name(w2454) -> ("ProjectName"=w2453:string, "AcutalOuput"=w2452:u32)
                n343 = Bundle("ProjectName"=w2453, "AcutalOuput"=w2452) -> (w2451:cluster{"ProjectName":string, "AcutalOuput":u32})  [unwired: 1 in]
                n344 = To Variant(anything=w2451) -> (Variant=w2456:variant)
                n345 = call "DB Update Data(Feedback).vi"("Pos"=cluster{"index":i32, "Len":i32} {"index"=1, "Len"=2}, "Sel index"=0, "data"=w2456, "error in (no error)"=w2463, "Code"=w2460, "table"=w2461, "Connncet State"=w2462) -> ("error out"=w2457:errorcluster, "State"=w2455:bool)  [unwired: 2 in, 1 out]
              }
            }
          }
        }
        n346 = call "Error cyc Times.vi"("error in (no error)"=w2409, "Status in"=w2410) -> ("error out"=w2402:errorcluster, "Numeric"=w2412:i32, "Cys Status"=w2411:bool)  [unwired: 6 in, 1 out]
        n347 = Equal?(x=w2412, y=2) -> (x = y?=w2414:bool)
        n348 = Select(t=string[] ["BR:Update AJ_EndRun", "Display Tip"], s=w2414, f=string[] ["BR:Update AJ_EndRun"]) -> (s? t:f=w2400:string[])
        n349 = Not(x=w2411) -> (.not. x?=w2401:bool)
      }
      frame "Display Tip" {
        n350 = Unbundle By Name(w2466) -> ("information"=w2465:T12)
        n351 = call "Log info.vi"("error in (no error)"=w2468, "information"=w2465) -> ("error out"=w2467:errorcluster)  [unwired: 8 in, 1 out]
      }
      frame "input & Ouput" {
        n352 = Unbundle By Name(w2475) -> ("Main.Ctr.Exit"=w2473:refnum<vi>)
        n353 = property class="Bool (严格)"(reference=w2473, error in=w2474) -> (error out=w2472:errorcluster, "Value"=w2471:bool)  [unwired: 1 out]
      }
      frame "Quit" {
      }
      frame "Error Log" {
        n354 = Unbundle By Name(w2487) -> ("information"=w2486:T12)
        n355 = Bundle By Name(cluster=w2486, "Status"=TRUE) -> (w2485:T12)
        n356 = call "Log info.vi"("error in (no error)"=w2490, "information"=w2485) -> ("error out"=w2489:errorcluster)  [unwired: 8 in, 1 out]
        n357 = call <vilib>:"Clear Errors.vi"("error in (no error)"=w2489) -> ("error out"=w2488:errorcluster)  [unwired: 5 in, 1 out]
        "Previous Event" <- w2482
      }
    }
    n358 = call "Insert Multiple Events(Error).vi"("error in (no error)"=w22, "Insert all? (T)"=w20, "Events to Insert"=w24, "Event queue in"=w25) -> ("error out"=w21:errorcluster, "Event queue out"=w26:string[])  [unwired: 6 in]
  }
  "error out" <- w11
